vi "Periodic Tasks.vi"(8 "error in":errorcluster) -> (0 "error out":errorcluster)   [LabVIEW 2018]
doc: "This VI runs in parallel to other tasks. It can contain as many user-defined periodic loops as you need. These can carry out PID or other sorts of timed response."
uses:
  <vilib>/Rock Robotics/WPI/Joystick/WPI_JoystickDevRef.ctl
  <vilib>/Rock Robotics/WPI/Joystick/WPI_JoystickDeviceEnum.ctl
  <vilib>/Rock Robotics/WPI/RobotDrive/WPI_RobotDriveDevRef.ctl
  <vilib>/Rock Robotics/WPI/MotorControl/WPI_MotorControlDeviceRef.ctl
  <vilib>/Rock Robotics/WPI/MotorControl/WPI_MotorControlType.ctl
  <vilib>/Rock Robotics/SystemInterfaces/DIO/FPGA_DIOPWMChannel.ctl
  <vilib>/Rock Robotics/WPI/PWM/WPI_PWMDeadband.ctl
  <vilib>/Rock Robotics/SystemInterfaces/DIO/FPGA_DIOChannel.ctl
  <vilib>/Rock Robotics/WPI/Solenoid/WPI_SolenoidDevRef.ctl
  <vilib>/Rock Robotics/WPI/Solenoid/WPI_SolenoidChannel.ctl
  <vilib>/Rock Robotics/WPI/DigitalInput/WPI_DigitalInputDevRef.ctl
  Vision States.ctl
  <vilib>/Rock Robotics/WPI/DriverStation/WPI_DriverStationRobotMode2.ctl
  Hatch Retainer States.ctl
  HAB Bk Spd Motor States.ctl
  Hatch Kicking States.ctl
  <vilib>/Rock Robotics/WPI/Solenoid/WPI_SolenoidValue.ctl
  <vilib>/Rock Robotics/WPI/ThirdParty/Phoenix-LabVIEW/Motor Controller/Controls/CTRE_Phoenix_MotorControl_ControlMode.ctl
  <vilib>/Rock Robotics/WPI/ThirdParty/Phoenix-LabVIEW/Motor Controller/Controls/CTRE_Phoenix_MotorControl_MotionProfileTrajectoryPoint.ctl
  <vilib>/Rock Robotics/WPI/Utilities/WPI_GetSetVariantRefNum.vi
  <vilib>/Rock Robotics/WPI/ThirdParty/Phoenix-LabVIEW/Motor Controller/Get/CTRE_Phoenix_MotorController_GetQuadratureData.vi
  Robot Global Data.vi
  <vilib>/Rock Robotics/Network Tables/NT Write Boolean.vi
  <vilib>/Rock Robotics/WPI/Solenoid/WPI_SolenoidSetEnum.vi
  <vilib>/addons/control/pid/pid.llb/PID (DBL).vi
  <vilib>/Rock Robotics/Network Tables/NT Write Number.vi
  <vilib>/Rock Robotics/WPI/ThirdParty/Phoenix-LabVIEW/Motor Controller/Closed Loop/Motion Profile/CTRE_Phoenix_MotorControl_BufferedTrajectoryPointStream_WriteAll.vi
  <vilib>/Rock Robotics/Network Tables/NT Read Number.vi
  <vilib>/addons/control/pid/NI_PID_pid.lvlib
panel:
  in  "HAB3DriveModuleMotorDevRef 2":T1={"DeviceStatus"={"status"=FALSE, "code"=0, "source"=""}, "Type"=enum."PWM", "PWM"={"PWM Channel"=enum."Invalid", "DeadBand"={"Name"="", "maxPositivePwm"=0, "minPositivePwm"=0, "centerPwm"=0, "maxNegativePwm"=0, "minNegativePwm"=0, "angularRange"=0}}, "CAN"={"Device Number"=0, "SetOutput VI Ref"=variant(refnum<vi> refnum), "GetOutput VI Ref"=variant(refnum<vi> refnum), "Enable VI Ref"=variant(refnum<vi> refnum), "Disable VI Ref"=variant(refnum<vi> refnum), "Data"=variant}, "Invert"=FALSE, "DIO PWM"={"PWM \"Enable\" Channel"=enum."Invalid", "DIOChannel"=enum."Invalid", "PWM Rate"=0.0}}
  in  "BkSpdAdjusterMotorDevRef":T1={"DeviceStatus"={"status"=FALSE, "code"=0, "source"=""}, "Type"=enum."PWM", "PWM"={"PWM Channel"=enum."Invalid", "DeadBand"={"Name"="", "maxPositivePwm"=0, "minPositivePwm"=0, "centerPwm"=0, "maxNegativePwm"=0, "minNegativePwm"=0, "angularRange"=0}}, "CAN"={"Device Number"=0, "SetOutput VI Ref"=variant(refnum<vi> refnum), "GetOutput VI Ref"=variant(refnum<vi> refnum), "Enable VI Ref"=variant(refnum<vi> refnum), "Disable VI Ref"=variant(refnum<vi> refnum), "Data"=variant}, "Invert"=FALSE, "DIO PWM"={"PWM \"Enable\" Channel"=enum."Invalid", "DIOChannel"=enum."Invalid", "PWM Rate"=0.0}}
  in  "HABAssisterSolenoidDevRef":T6={"DevStatus"={"status"=FALSE, "code"=0, "source"=""}, "Pneumatics Control Module"=0, "Forward Solenoid Channel"=enum."Invalid", "Reverse Solenoid Channel"=enum."Invalid"}
  out "Right Traj. Pts Array":dbl[][](array[numeric])
  out "Left Traj. Pts Array":dbl[][](array[numeric])
  in  "Back HAB 3 Limit Switch":T8={"DevStatus"={"status"=FALSE, "code"=0, "source"=""}, "DIO Channel"=enum."Invalid"}
  in  "Front HAB 3 Limit Switch":T8={"DevStatus"={"status"=FALSE, "code"=0, "source"=""}, "DIO Channel"=enum."Invalid"}
  in  "BottomRetainerSwitchDevRef":T8={"DevStatus"={"status"=FALSE, "code"=0, "source"=""}, "DIO Channel"=enum."Invalid"}
  in  "TopRetainerSwitchDevRef":T8={"DevStatus"={"status"=FALSE, "code"=0, "source"=""}, "DIO Channel"=enum."Invalid"}
  in  "HatchRetainerMotorDevRef":T1={"DeviceStatus"={"status"=FALSE, "code"=0, "source"=""}, "Type"=enum."PWM", "PWM"={"PWM Channel"=enum."Invalid", "DeadBand"={"Name"="", "maxPositivePwm"=0, "minPositivePwm"=0, "centerPwm"=0, "maxNegativePwm"=0, "minNegativePwm"=0, "angularRange"=0}}, "CAN"={"Device Number"=0, "SetOutput VI Ref"=variant(refnum<vi> refnum), "GetOutput VI Ref"=variant(refnum<vi> refnum), "Enable VI Ref"=variant(refnum<vi> refnum), "Disable VI Ref"=variant(refnum<vi> refnum), "Data"=variant}, "Invert"=FALSE, "DIO PWM"={"PWM \"Enable\" Channel"=enum."Invalid", "DIOChannel"=enum."Invalid", "PWM Rate"=0.0}}
  in  "HAB3BackSolenoidDevRef":T6={"DevStatus"={"status"=FALSE, "code"=0, "source"=""}, "Pneumatics Control Module"=0, "Forward Solenoid Channel"=enum."Invalid", "Reverse Solenoid Channel"=enum."Invalid"}
  in  "HAB3FrontSolenoidDevRef":T6={"DevStatus"={"status"=FALSE, "code"=0, "source"=""}, "Pneumatics Control Module"=0, "Forward Solenoid Channel"=enum."Invalid", "Reverse Solenoid Channel"=enum."Invalid"}
  in  "AuxJoystickDevRef":T9={"Device"=enum."USB 1"}
  in  "DriveJoystickDevRef":T9={"Device"=enum."USB 1"}
  in  "HAB3DriveModuleMotorDevRef":T1={"DeviceStatus"={"status"=FALSE, "code"=0, "source"=""}, "Type"=enum."PWM", "PWM"={"PWM Channel"=enum."Invalid", "DeadBand"={"Name"="", "maxPositivePwm"=0, "minPositivePwm"=0, "centerPwm"=0, "maxNegativePwm"=0, "minNegativePwm"=0, "angularRange"=0}}, "CAN"={"Device Number"=0, "SetOutput VI Ref"=variant(refnum<vi> refnum), "GetOutput VI Ref"=variant(refnum<vi> refnum), "Enable VI Ref"=variant(refnum<vi> refnum), "Disable VI Ref"=variant(refnum<vi> refnum), "Data"=variant}, "Invert"=FALSE, "DIO PWM"={"PWM \"Enable\" Channel"=enum."Invalid", "DIOChannel"=enum."Invalid", "PWM Rate"=0.0}}
  in  "LifterSolenoidDevRef":T6={"DevStatus"={"status"=FALSE, "code"=0, "source"=""}, "Pneumatics Control Module"=0, "Forward Solenoid Channel"=enum."Invalid", "Reverse Solenoid Channel"=enum."Invalid"}
  in  "DriveJoystickDevRef":T9={"Device"=enum."USB 1"}
  in  "HatchCollectorMotorDevRef":T1={"DeviceStatus"={"status"=FALSE, "code"=0, "source"=""}, "Type"=enum."PWM", "PWM"={"PWM Channel"=enum."Invalid", "DeadBand"={"Name"="", "maxPositivePwm"=0, "minPositivePwm"=0, "centerPwm"=0, "maxNegativePwm"=0, "minNegativePwm"=0, "angularRange"=0}}, "CAN"={"Device Number"=0, "SetOutput VI Ref"=variant(refnum<vi> refnum), "GetOutput VI Ref"=variant(refnum<vi> refnum), "Enable VI Ref"=variant(refnum<vi> refnum), "Disable VI Ref"=variant(refnum<vi> refnum), "Data"=variant}, "Invert"=FALSE, "DIO PWM"={"PWM \"Enable\" Channel"=enum."Invalid", "DIOChannel"=enum."Invalid", "PWM Rate"=0.0}}
  in  "AuxJoystickDevRef":T9
  in  "RetainerSolenoidDevRef":T6={"DevStatus"={"status"=FALSE, "code"=0, "source"=""}, "Pneumatics Control Module"=0, "Forward Solenoid Channel"=enum."Invalid", "Reverse Solenoid Channel"=enum."Invalid"}
  in  "KickerSolenoidDevRef":T6={"DevStatus"={"status"=FALSE, "code"=0, "source"=""}, "Pneumatics Control Module"=0, "Forward Solenoid Channel"=enum."Invalid", "Reverse Solenoid Channel"=enum."Invalid"}
  in  "Drive Motors":T11={"DevStatus"={"status"=FALSE, "code"=0, "source"=""}, "Motors[]"=[], "Square Inputs"=FALSE, "Max Output"=1.0}
  in  "AuxJoystickDevRef":T9={"Device"=enum."USB 1"}
  in  "DriveJoystickDevRef":T9
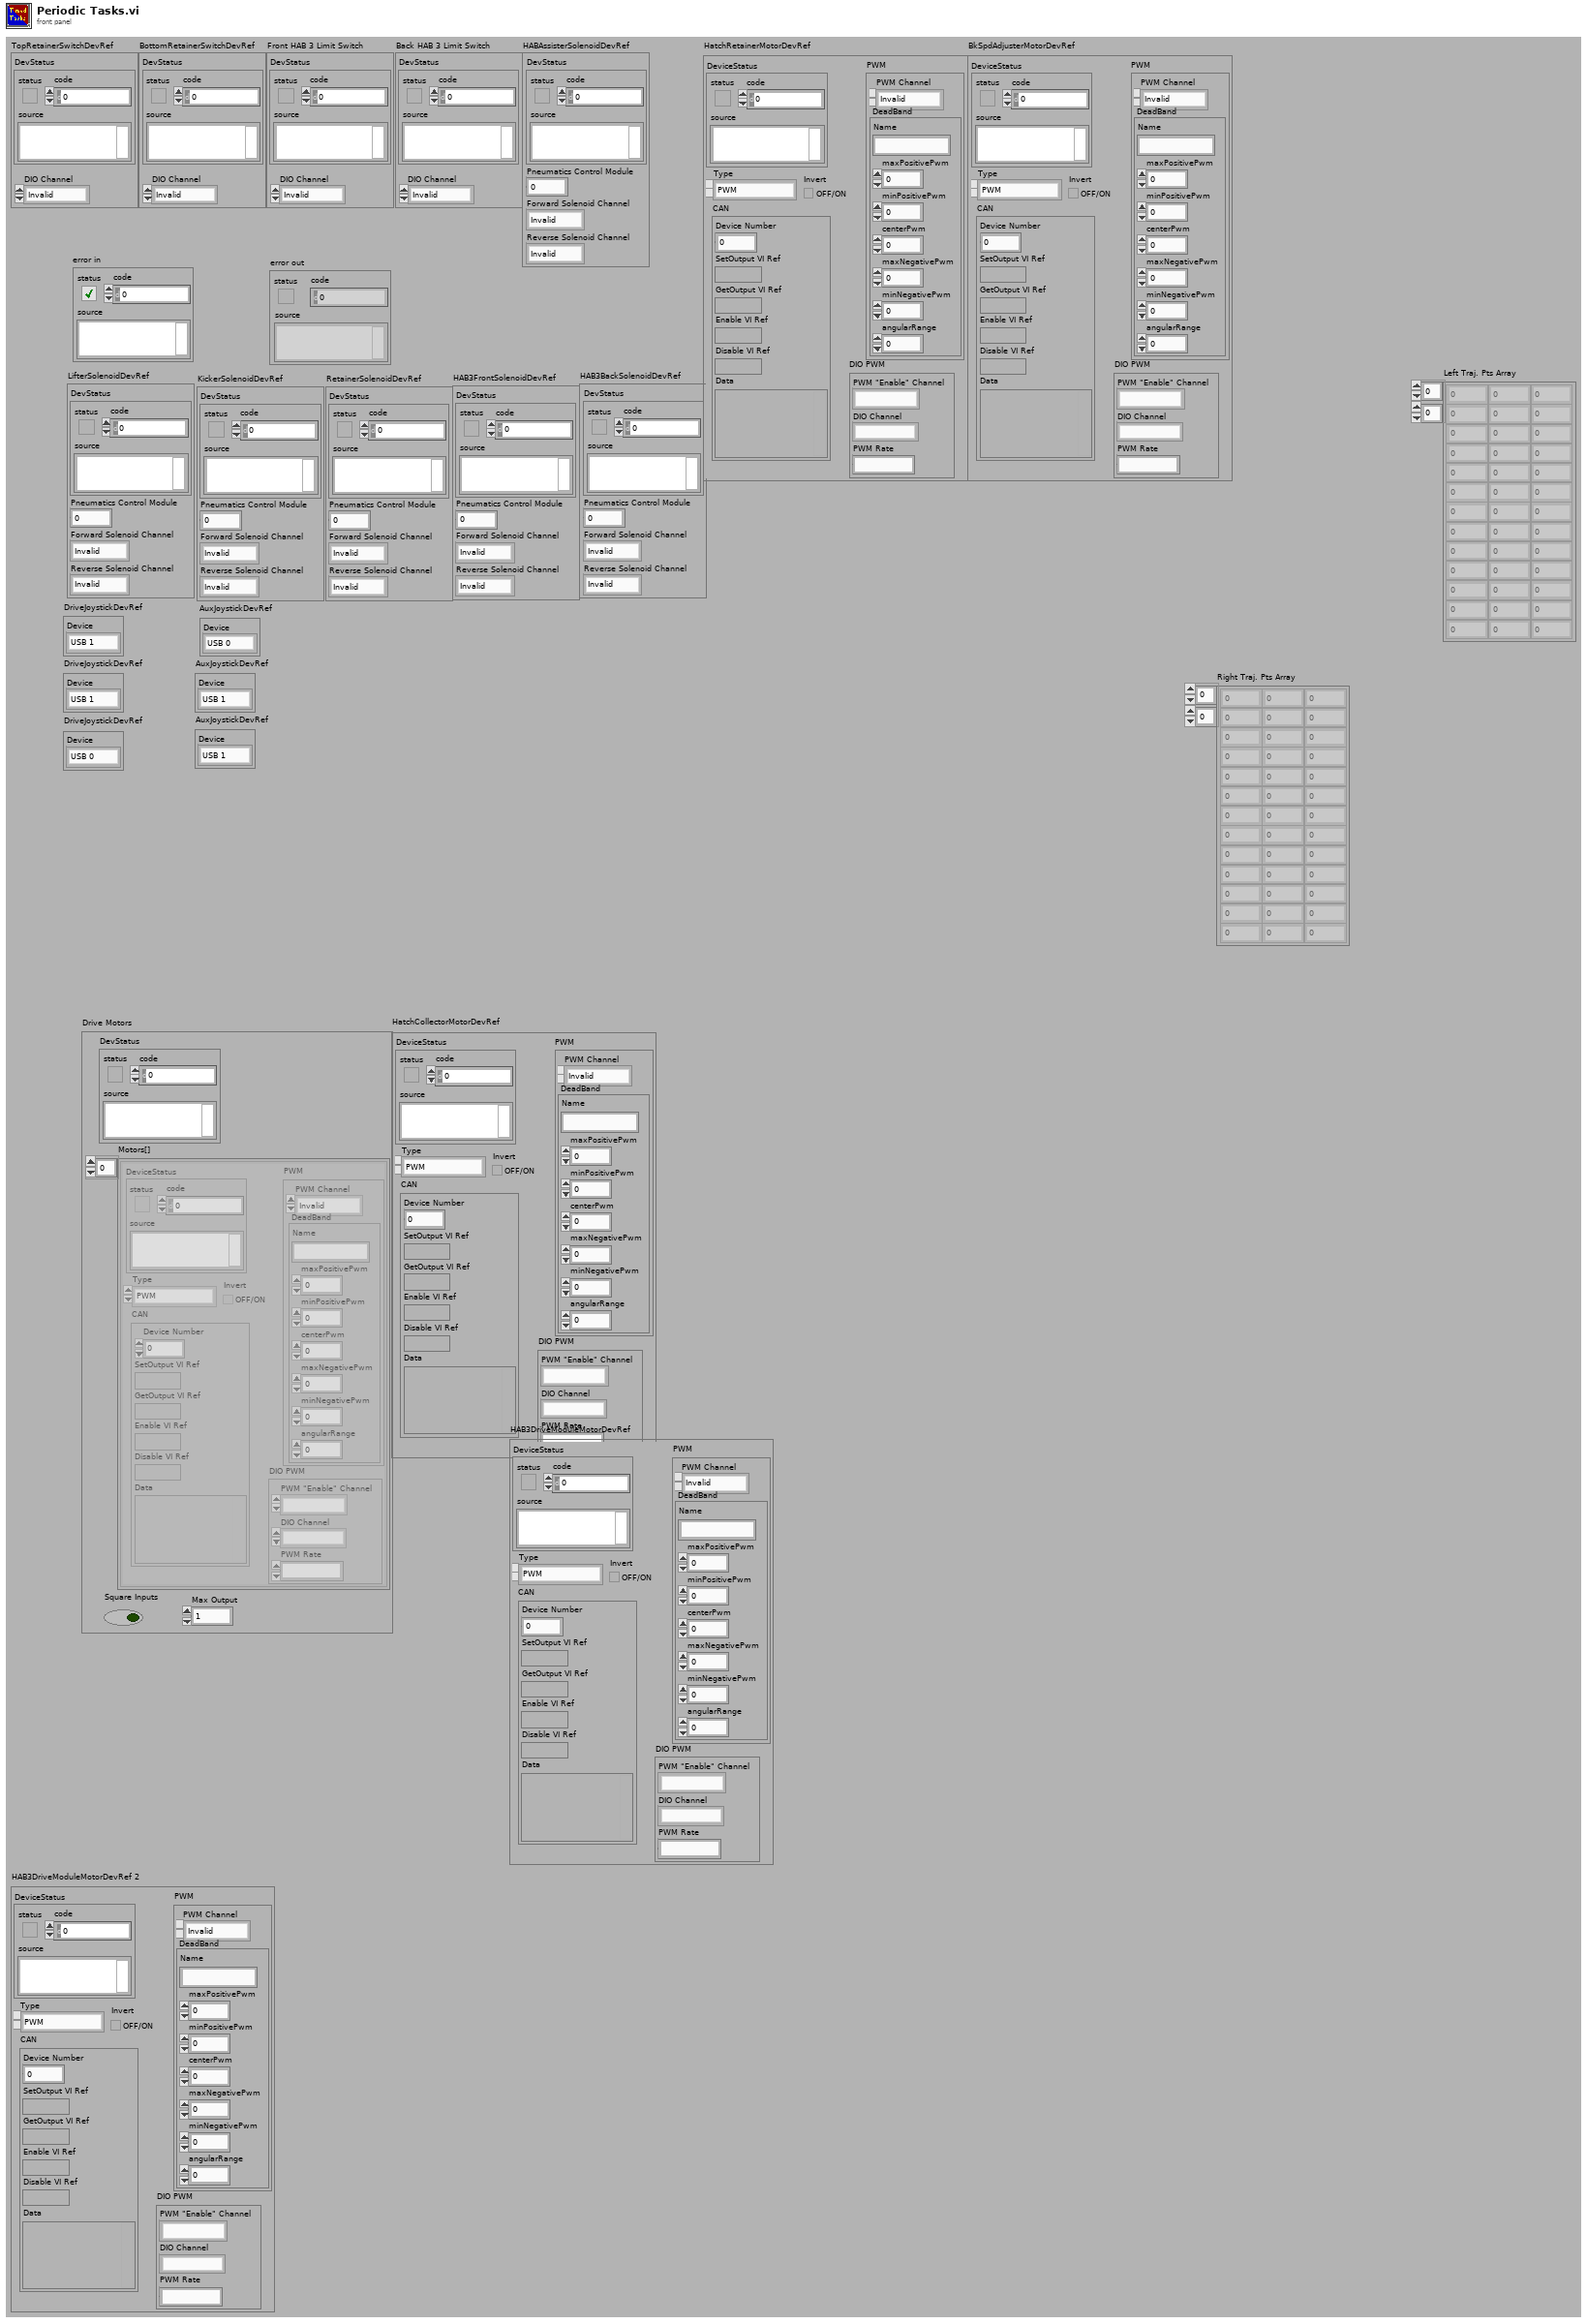
[diagram p1: front panel]
types:
  T1 = typedef "WPI_MotorControlDeviceRef.ctl" = cluster{"DeviceStatus":errorcluster, "Type":T2, "PWM":cluster{"PWM Channel":T3, "DeadBand":T4}, "CAN":cluster{"Device Number":u8, "SetOutput VI Ref":variant, "GetOutput VI Ref":variant, "Enable VI Ref":variant, "Disable VI Ref":variant, "Data":variant}, "Invert":bool, "DIO PWM":cluster{"PWM \"Enable\" Channel":T3, "DIOChannel":T5, "PWM Rate":dbl}}
  T2 = typedef "WPI_MotorControlType.ctl" = enum16{"PWM", "CAN", "DIO PWM"}
  T3 = typedef "FPGA_DIOPWMChannel.ctl" = enum8{"PWM 0", "PWM 1", "PWM 2", "PWM 3", "PWM 4", "PWM 5", "PWM 6", "PWM 7", "PWM 8", "PWM 9", "PWM MXP 0", "PWM MXP 1", "PWM MXP 2", "PWM MXP 3", "PWM MXP 4", "PWM MXP 5", "PWM MXP 6", "PWM MXP 7", "PWM MXP 8", "PWM MXP 9", "Invalid"}
  T4 = typedef "WPI_PWMDeadband.ctl" = cluster{"Name":string, "maxPositivePwm":i32, "minPositivePwm":i32, "centerPwm":i32, "maxNegativePwm":i32, "minNegativePwm":i32, "angularRange":u16}
  T5 = typedef "FPGA_DIOChannel.ctl" = enum8{"DIO 0", "DIO 1", "DIO 2", "DIO 3", "DIO 4", "DIO 5", "DIO 6", "DIO 7", "DIO 8", "DIO 9", "DIO MXP 0", "DIO MXP 1", "DIO MXP 2", "DIO MXP 3", "DIO MXP 4", "DIO MXP 5", "DIO MXP 6", "DIO MXP 7", "DIO MXP 8", "DIO MXP 9", "DIO MXP 10", "DIO MXP 11", "DIO MXP 12", "DIO MXP 13", "DIO MXP 14", "DIO MXP 15", "SPI Port CS1", "SPI Port CS2", "SPI Port CS3", "SPI Port MISO", "SPI Port MOSI", "Invalid"}
  T6 = typedef "WPI_SolenoidDevRef.ctl" = cluster{"DevStatus":errorcluster, "Pneumatics Control Module":u8, "Forward Solenoid Channel":T7, "Reverse Solenoid Channel":T7}
  T7 = typedef "WPI_SolenoidChannel.ctl" = enum8{"Solenoid 0", "Solenoid 1", "Solenoid 2", "Solenoid 3", "Solenoid 4", "Solenoid 5", "Solenoid 6", "Solenoid 7", "Invalid"}
  T8 = typedef "WPI_DigitalInputDevRef.ctl" = cluster{"DevStatus":errorcluster, "DIO Channel":T5}
  T9 = typedef "WPI_JoystickDevRef.ctl" = cluster{"Device":T10}
  T10 = typedef "WPI_JoystickDeviceEnum.ctl" = enum16{"USB 0", "USB 1", "USB 2", "USB 3", "USB 4", "USB 5"}
  T11 = typedef "WPI_RobotDriveDevRef.ctl" = cluster{"DevStatus":errorcluster, "Motors[]":T1[], "Square Inputs":bool, "Max Output":dbl}
  T12 = typedef "Hatch Kicking States.ctl" = enum16{"Ready", "Stop Retaining Hatch", "Kick Hatch"}
  T13 = typedef "HAB Bk Spd Motor States.ctl" = enum16{"Fully Up", "Going Down", "Fully Down", "Going Up"}
  T14 = typedef "Hatch Retainer States.ctl" = enum16{"Fully Down (not retained)", "Going Up", "Fully Up (retained)", "Going Down"}
  T15 = cluster{"X Button":i32, "A Button":i32, "B Button":i32, "Y Button":i32, "LB Button":i32, "RB Button":i32, "LT Button":i32, "RT Button":i32, "BACK Button":i32, "START Button":i32, "LJ Click Button":i32, "RJ Click Button":i32}
  T16 = cluster{"Left X":i32, "Left Y":i32, "Right X":i32, "Right Y":i32}
  T17 = typedef "WPI_DriverStationRobotMode2.ctl" = enum16{"Autonomous Disabled", "Autonomous Enabled", "Teleop Disabled", "Teleop Enabled", "Disconnected", "Finish", "Test Disabled", "Test Enabled", "Emergency Stopped"}
  T18 = cluster{"offsetAngle H":dbl, "offsetAngle V":dbl, "area":dbl, "skew":dbl, "shortest side (pxls)":dbl, "longest side (pxls)":dbl}
  T19 = typedef "Vision States.ctl" = enum16{"Ready", "Forward Until Target at Edge", "Vision Track"}
  T20 = cluster{"A Button":i32, "B Button":i32, "X Button":i32, "Y Button":i32, "LB Button":i32, "RB Button":i32, "BACK Button":i32, "START Button":i32, "LJ Click Button":i32, "RJ Click Button":i32}
  T21 = cluster{"Left X":i32, "Left Y":i32, "Right X":i32, "Right Y":i32, "RT Button":i32, "LT Button":i32}
  T22 = typedef "WPI_GyroDevRef.ctl" = cluster{"DevStatus":errorcluster, "Analog Channel":T23, "Gain (VoltsPerDegree/Second)":dbl, "Gyro Type":enum16{"Analog", "XRS450"}, "Handle":i32, "SPI Bus":T24, "Device Found":bool, "Sample Rate":dbl, "Calibrate On Open":bool, "Offset":dbl}
  T23 = typedef "FPGA_AIChannel.ctl" = enum8{"AI 0", "AI 1", "AI 2", "AI 3", "AI MXP 0", "AI MXP 1", "AI MXP 2", "AI MXP 3", "Invalid"}
  T24 = typedef "spi_bus.ctl" = enum16{"SPI On-Board, CS0", "SPI On-Board, CS1", "SPI On-Board, CS2", "SPI On-Board, CS3", "SPI MXP", "Invalid"}
  T25 = cluster{"HAB3DriveModuleMotorDevRef 2":T1, "DriveJoystickDevRef":T9, "AuxJoystickDevRef":T9, "Drive Axes":dbl[], "Drive Buttons":bool[], "Drive POVs":i16[], "Aux Axes":dbl[], "Aux Buttons":bool[], "Aux POVs":i16[], "Robot Mode":T17, "Drive Motors":T11, "Drive Axes Indexes":cluster{"Left X":i32, "Left Y":i32, "Right X":i32, "Right Y":i32, "RT Button":i32, "LT Button":i32}, "Drive Button Indexes":cluster{"A Button":i32, "B Button":i32, "X Button":i32, "Y Button":i32, "LB Button":i32, "RB Button":i32, "BACK Button":i32, "START Button":i32, "LJ Click Button":i32, "RJ Click Button":i32}, "Joystick VS Vision Latch":bool, "Vision States":T19, "limelight":cluster{"offsetAngle H":dbl, "offsetAngle V":dbl, "area":dbl, "skew":dbl, "shortest side (pxls)":dbl, "longest side (pxls)":dbl}, "Vision Track Mode Override":bool, "T = Motion Profile, F = Percent Output":bool, "Arcade Drive?":bool, "Start Motion Profile?":bool}
  T26 = cluster{"TopRetainerSwitchDevRef":T8, "BottomRetainerSwitchDevRef":T8, "HatchRetainerMotorDevRef":T1, "LifterSolenoidDevRef":T6, "DriveJoystickDevRef":T9, "KickerSolenoidDevRef":T6, "RetainerSolenoidDevRef":T6, "AuxJoystickDevRef":T9, "HatchCollectorMotorDevRef":T1, "Drive Axes":dbl[], "Drive Buttons":bool[], "Drive POVs":i16[], "Aux Axes":dbl[], "Aux Buttons":bool[], "Aux POVs":i16[], "Robot Mode":T17, "Aux Joystick Indexes":cluster{"Left X":i32, "Left Y":i32, "Right X":i32, "Right Y":i32}, "Aux Button Indexes":cluster{"X Button":i32, "A Button":i32, "B Button":i32, "Y Button":i32, "LB Button":i32, "RB Button":i32, "LT Button":i32, "RT Button":i32, "BACK Button":i32, "START Button":i32, "LJ Click Button":i32, "RJ Click Button":i32}, "Hatch Retainer Move Up/Down":bool, "Hatch Collector Actual Angle":dbl, "Hatch Collector Wanted Angle":dbl, "Hatch Retainer States":T14, "Hatch Kicking States":T12}
  T27 = cluster{"BkSpdAdjusterMotorDevRef":T1, "HABAssisterSolenoidDevRef":T6, "Back HAB 3 Limit Switch":T8, "Front HAB 3 Limit Switch":T8, "HAB3DriveModuleMotorDevRef":T1, "DriveJoystickDevRef":T9, "AuxJoystickDevRef":T9, "HAB3FrontSolenoidDevRef":T6, "HAB3BackSolenoidDevRef":T6, "Drive Axes":dbl[], "Drive Buttons":bool[], "Drive POVs":i16[], "Aux Axes":dbl[], "Aux Buttons":bool[], "Aux POVs":i16[], "Robot Mode":T17, "Aux Joystick Indexes":cluster{"Left X":i32, "Left Y":i32, "Right X":i32, "Right Y":i32}, "Aux Button Indexes":cluster{"X Button":i32, "A Button":i32, "B Button":i32, "Y Button":i32, "LB Button":i32, "RB Button":i32, "LT Button":i32, "RT Button":i32, "BACK Button":i32, "START Button":i32, "LJ Click Button":i32, "RJ Click Button":i32}, "Front Cylinders Latch":bool, "Back Cylinders Latch":bool, "Yaw":dbl, "Pitch":dbl, "Roll":dbl, "HAB Bk Spd Motor States":T13}
  T28 = typedef "CTRE_Phoenix_MotorControl_MotionProfileTrajectoryPoint.ctl" = cluster{"Position":dbl, "Velocity":dbl, "Arbitrary Feed Forward":dbl, "Auxiliary Position":dbl, "Auxiliary Velocity":dbl, "Auxiliary Arbitrary Feed Forward":dbl, "Profile Slot Select":i32, "Auxiliary Profile Slot Select":i32, "isLastPoint?":bool, "Zero Position?":bool, "durationMs":u32, "Use Aux PID?":bool}
  T29 = typedef "Which Robot Enum.ctl" = enum16{"Competition Bot", "Practice Bot", "Code Bot"}
  T30 = typedef "CTRE_Phoenix_MotorControl_BufferedTrajectoryPointStream_DeviceRef.ctl" = cluster{"Handle":u64, "Library Path":path}
  T31 = typedef "WPI_SolenoidValue.ctl" = enum16{"Off", "On", "Forward", "Reverse"}
  T32 = cluster{"proportional gain (Kc)":dbl, "integral time (Ti, min)":dbl, "derivative time (Td, min)":dbl}
  T33 = typedef "CTRE_Phoenix_MotorControl_ControlMode.ctl" = u16
  T34 = cluster{"Yaw":dbl, "Roll":dbl, "Pitch":dbl, "Heading":dbl, "Fused Heading":dbl}
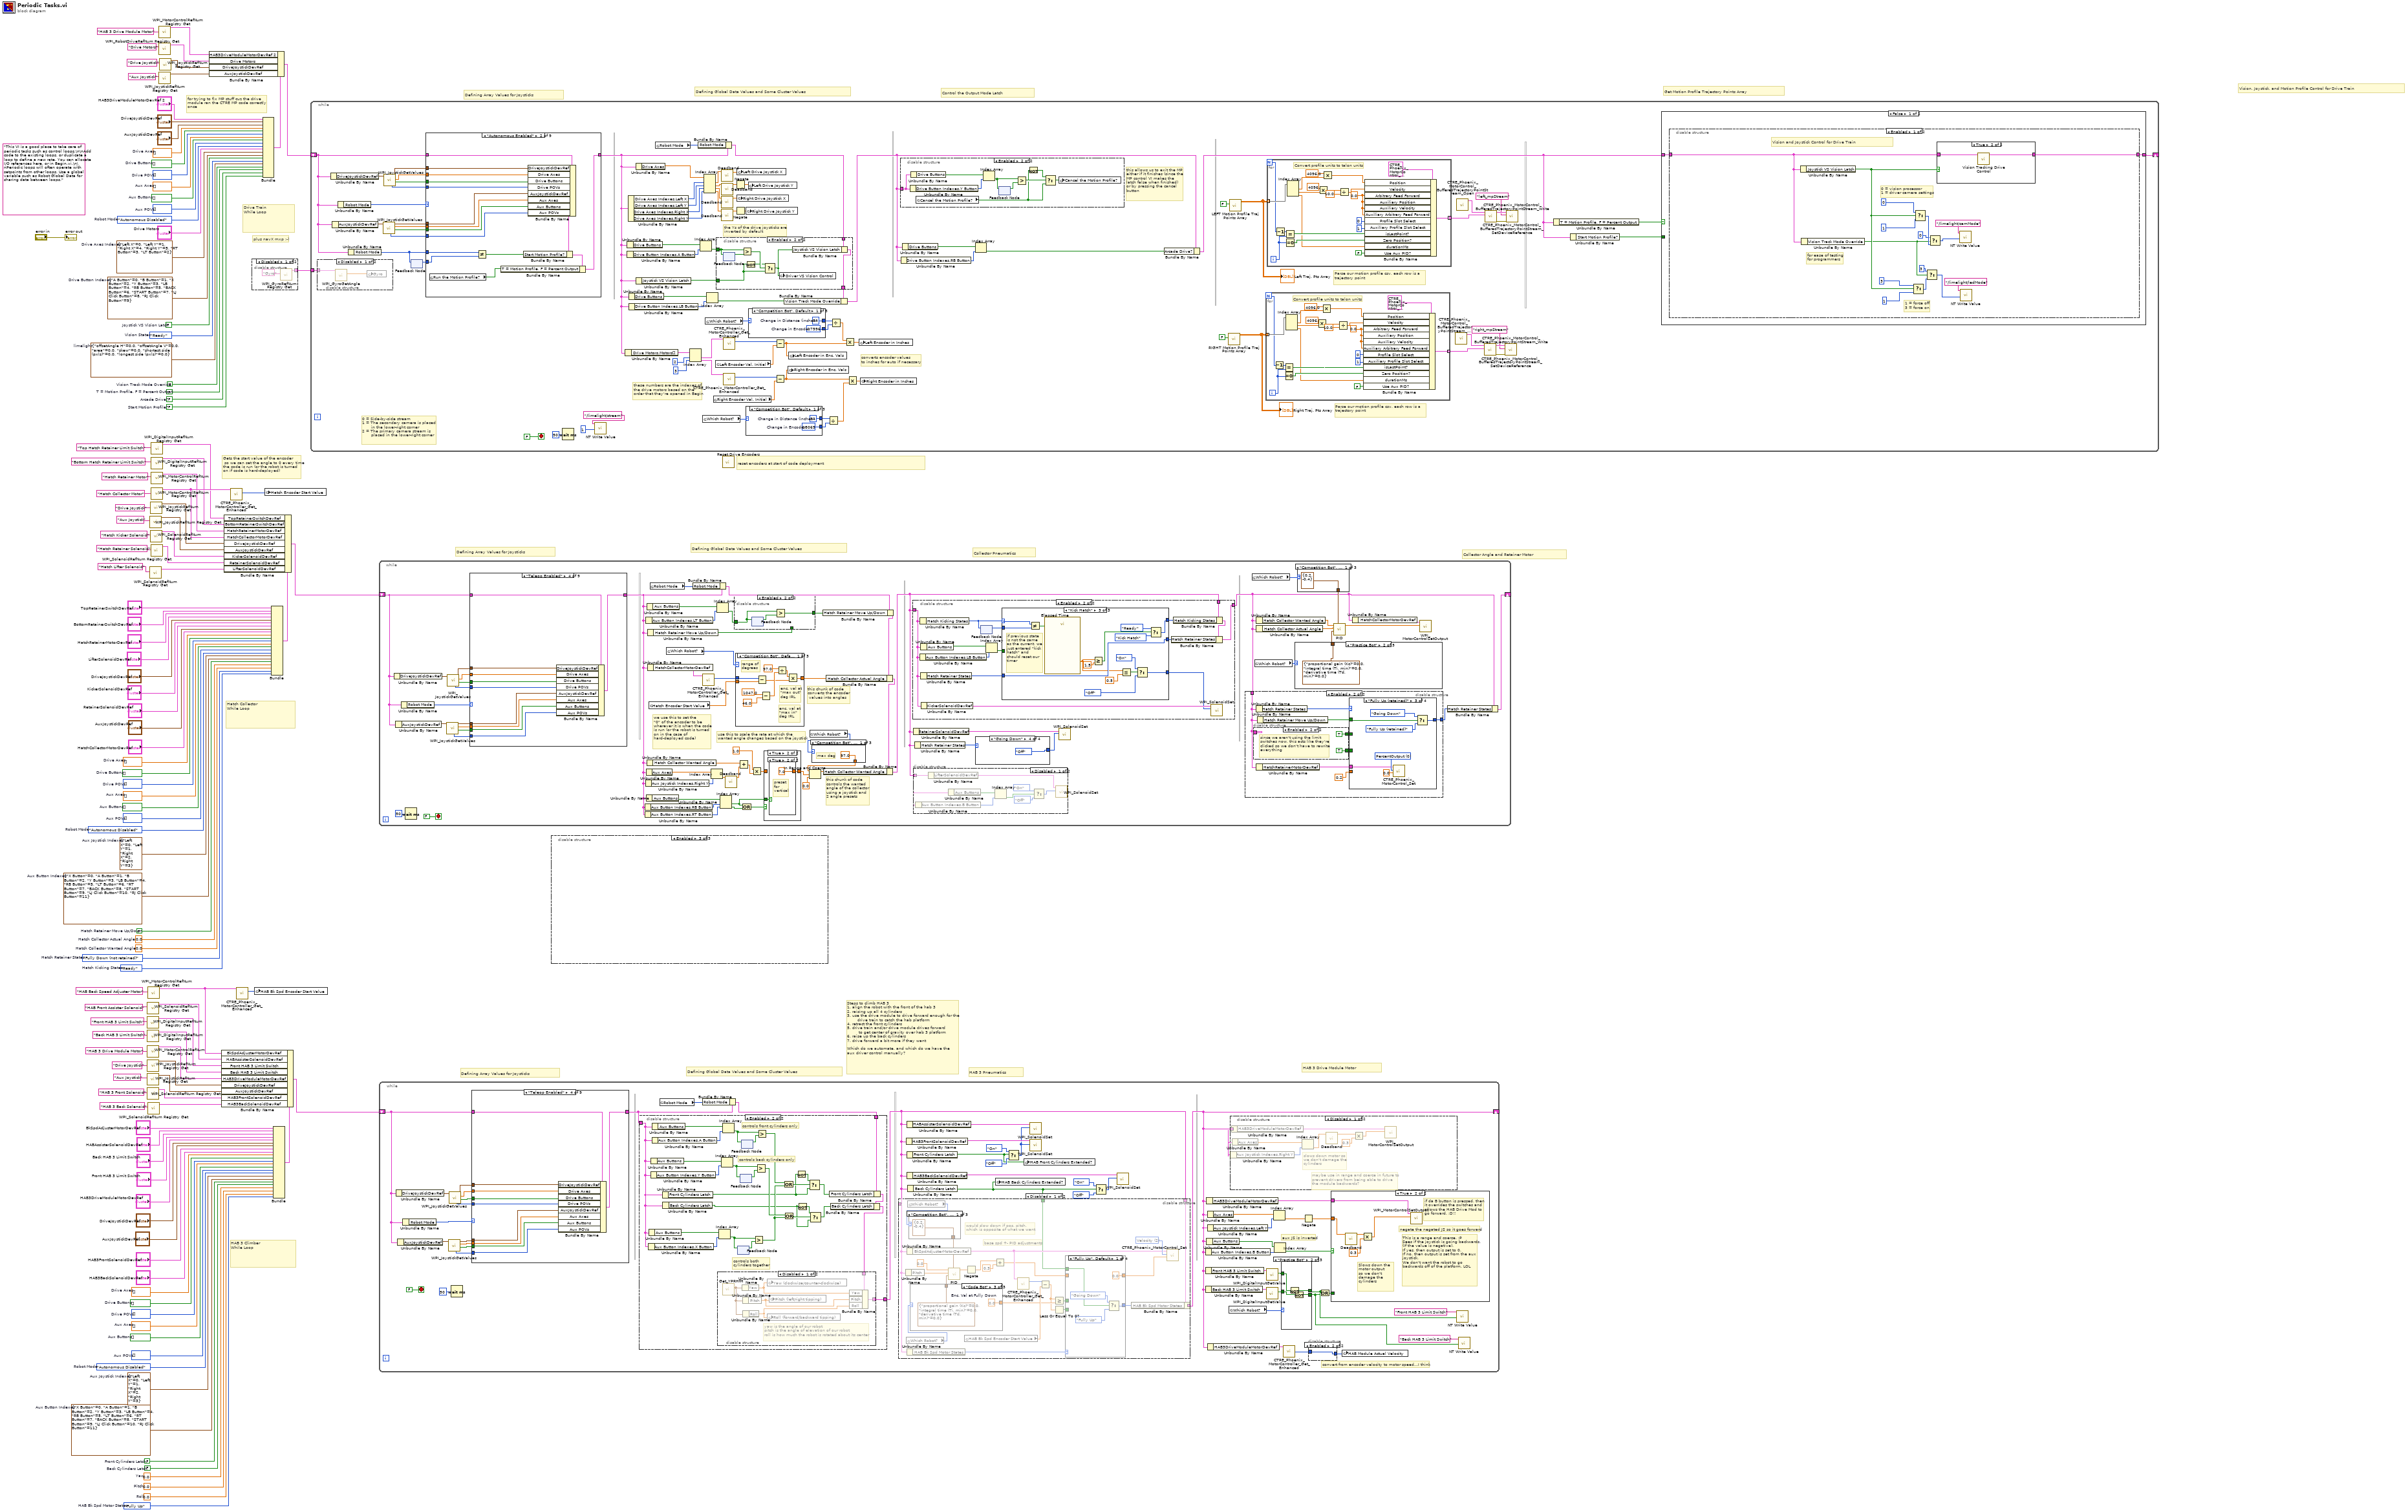
[diagram p0: block diagram]
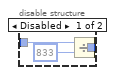
[diagram p2: hidden frame]
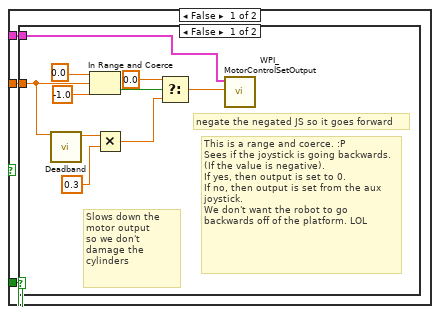
[diagram p3: hidden frame]
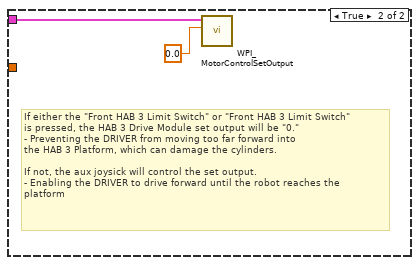
[diagram p4: hidden frame]
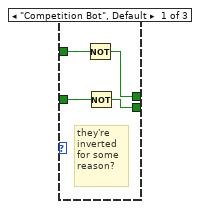
[diagram p5: hidden frame]
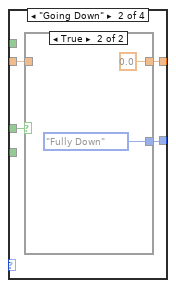
[diagram p7: hidden frame]
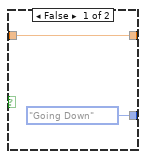
[diagram p8: hidden frame]
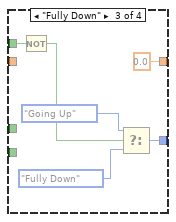
[diagram p9: hidden frame]
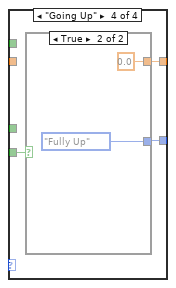
[diagram p10: hidden frame]
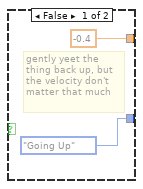
[diagram p11: hidden frame]
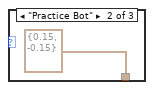
[diagram p12: hidden frame]
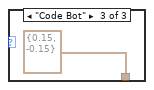
[diagram p13: hidden frame]
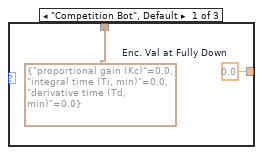
[diagram p14: hidden frame]
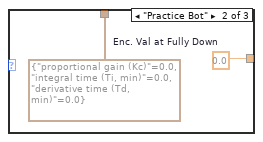
[diagram p15: hidden frame]
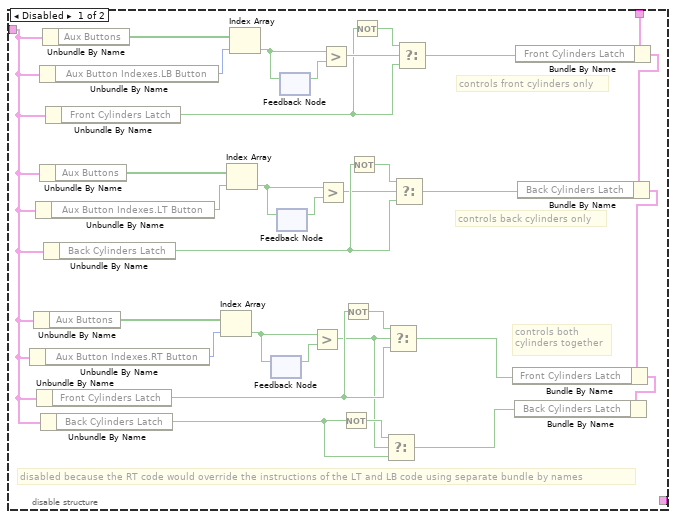
[diagram p17: hidden frame]
diagram:
  w4 = FALSE  # Start Motion Profile?
  w5 = FALSE  # Arcade Drive?
  w6 = Hatch_Kicking_States."Ready"  # Hatch Kicking States
  w7 = HAB_Bk_Spd_Motor_States."Fully Up"  # HAB Bk Spd Motor States
  w12 = 0.0  # Roll
  w13 = 0.0  # Pitch
  w14 = 0.0  # Yaw
  w24 = Hatch_Retainer_States."Fully Down (not retained)"  # Hatch Retainer States
  w34 = FALSE  # T = Motion Profile, F = Percent Output
  w36 = 0.0  # Hatch Collector Wanted Angle
  w37 = FALSE  # Back Cylinders Latch
  w38 = FALSE  # Front Cylinders Latch
  w39 = T15 {"X Button"=0, "A Button"=1, "B Button"=2, "Y Button"=3, "LB Button"=4, "RB Button"=5, "LT Button"=6, "RT Button"=7, "BACK Button"=8, "START Button"=9, "LJ Click Button"=10, "RJ Click Button"=11}  # Aux Button Indexes
  w40 = T16 {"Left X"=0, "Left Y"=1, "Right X"=2, "Right Y"=3}  # Aux Joystick Indexes
  w41 = WPI_DriverStationRobotMode2."Autonomous Disabled"  # Robot Mode
  w42 = i16[] []  # Aux POVs
  w43 = bool[] []  # Aux Buttons
  w44 = dbl[] []  # Aux Axes
  w45 = i16[] []  # Drive POVs
  w46 = bool[] []  # Drive Buttons
  w47 = dbl[] []  # Drive Axes
  w70 = 0.0  # Hatch Collector Actual Angle
  w71 = FALSE  # Hatch Retainer Move Up/Down
  w72 = T15 {"X Button"=0, "A Button"=1, "B Button"=2, "Y Button"=3, "LB Button"=4, "RB Button"=5, "LT Button"=6, "RT Button"=7, "BACK Button"=8, "START Button"=9, "LJ Click Button"=10, "RJ Click Button"=11}  # Aux Button Indexes
  w73 = T16 {"Left X"=0, "Left Y"=1, "Right X"=2, "Right Y"=3}  # Aux Joystick Indexes
  w77 = WPI_DriverStationRobotMode2."Autonomous Disabled"  # Robot Mode
  w78 = i16[] []  # Aux POVs
  w79 = bool[] []  # Aux Buttons
  w80 = dbl[] []  # Aux Axes
  w81 = i16[] []  # Drive POVs
  w82 = bool[] []  # Drive Buttons
  w83 = dbl[] []  # Drive Axes
  w97 = FALSE  # Vision Track Mode Override
  w98 = T18 {"offsetAngle H"=0.0, "offsetAngle V"=0.0, "area"=0.0, "skew"=0.0, "shortest side (pxls)"=0.0, "longest side (pxls)"=0.0}  # limelight
  w99 = Vision_States."Ready"  # Vision States
  w100 = FALSE  # Joystick VS Vision Latch
  w101 = T20 {"A Button"=0, "B Button"=1, "X Button"=2, "Y Button"=3, "LB Button"=4, "RB Button"=5, "BACK Button"=6, "START Button"=7, "LJ Click Button"=8, "RJ Click Button"=9}  # Drive Button Indexes
  w103 = T21 {"Left X"=0, "Left Y"=1, "Right X"=4, "Right Y"=5, "RT Button"=3, "LT Button"=2}  # Drive Axes Indexes
  w108 = i16[] []  # Aux POVs
  w109 = bool[] []  # Aux Buttons
  w110 = dbl[] []  # Aux Axes
  w107 = WPI_DriverStationRobotMode2."Autonomous Disabled"  # Robot Mode
  w111 = i16[] []  # Drive POVs
  w112 = bool[] []  # Drive Buttons
  w113 = dbl[] []  # Drive Axes
  (unwired) "This VI is a good place to take care of periodic tasks such as control loops.\n\nAdd code to the existing loops, or duplicate a loop to define a new rate. You can allocate I/O references here, or in Begin.vi.\n\nPeriodic loops will often operate with setpoints from other loops. Use a global variable such as Robot Global Data for sharing data between loops."
  # "HAB 3 Drive Module Motor"
  # "HAB 3 Pneumatics"
  # "Steps to climb HAB 3\n1. align the robot with the front of the hab 3\n2. raising up all 4 cylinders\n3. use the drive module to drive forward enough for the \n        drive train to catch the hab platform\n4. retract the front cylinders\n5. drive train and/or drive module drives forward \n         to get center of gravity over hab 3 platform\n6. raise up the back cylinders\n7. drive forward a bit more if they want\n\nWhich do we automate, and which do we have the \naux driver control manually?"
  # "Defining Global Data Values and Some Cluster Values"
  # "Defining Array Values for Joysticks"
  # "Collector Angle and Retainer Motor"
  # "Collector Pneumatics"
  # "Defining Global Data Values and Some Cluster Values"
  # "Defining Array Values for Joysticks"
  # "for trying to fix MP stuff cuz the drive\nmodule ran the CTRE MP code correctly\nonce"
  # "reset encoders at start of code deployment"
  # "Get Motion Profile Trajectory Points Array"
  # "Control the Output Mode Latch"
  # "plus navX mxp :-)"
  # "Gets the start value of the encoder\n so we can set the angle to 0 every time\nthe code is run (or the robot is turned\non if code is hard-deployed)"
  # "HAB 3 Climber\nWhile Loop"
  # "Hatch Collector\nWhile Loop"
  # "Drive Train\nWhile Loop"
  # "Vision, Joystick, and Motion Profile Control for Drive Train"
  # "Defining Array Values for Joysticks"
  # "Defining Global Data Values and Some Cluster Values"
  n1 = call <vilib>:"WPI_DigitalInputRefNum Registry Get.vi"("refnum name"="Front HAB 3 Limit Switch") -> ("DigitalInputDevRef"=w19:T8)  [unwired: 9 in, 1 out]
  n2 = call <vilib>:"WPI_JoystickRefNum Registry Get.vi"("refnum name"="Aux Joystick") -> ("JoystickDevRef"=w51:T9)  [unwired: 9 in, 1 out]
  n3 = call <vilib>:"WPI_SolenoidRefNum Registry Get.vi"("refnum name"="HAB Front Assister Solenoid") -> ("SolenoidDevRef"=w15:T6)  [unwired: 9 in, 1 out]
  n4 = call <vilib>:"WPI_DigitalInputRefNum Registry Get.vi"("refnum name"="Back HAB 3 Limit Switch") -> ("DigitalInputDevRef"=w18:T8)  [unwired: 9 in, 1 out]
  n5 = call <vilib>:"WPI_MotorControlRefNum Registry Get.vi"("refnum name"="HAB 3 Drive Module Motor") -> ("MotorControlDevRef"=w49:T1)  [unwired: 9 in, 1 out]
  n6 = call <vilib>:"WPI_JoystickRefNum Registry Get.vi"("refnum name"="Drive Joystick") -> ("JoystickDevRef"=w50:T9)  [unwired: 9 in, 1 out]
  n7 = call <vilib>:"WPI_SolenoidRefNum Registry Get.vi"("refnum name"="HAB 3 Front Solenoid") -> ("SolenoidDevRef"=w52:T6)  [unwired: 9 in, 1 out]
  n8 = call <vilib>:"WPI_MotorControlRefNum Registry Get.vi"("refnum name"="HAB Back Speed Adjuster Motor") -> ("MotorControlDevRef"=w8:T1)  [unwired: 9 in, 1 out]
  n9 = call <vilib>:"WPI_SolenoidRefNum Registry Get.vi"("refnum name"="HAB 3 Back Solenoid") -> ("SolenoidDevRef"=w53:T6)  [unwired: 9 in, 1 out]
  n10 = call <vilib>:"WPI_SolenoidRefNum Registry Get.vi"("refnum name"="Hatch Lifter Solenoid") -> ("SolenoidDevRef"=w66:T6)  [unwired: 9 in, 1 out]
  n11 = call <vilib>:"WPI_JoystickRefNum Registry Get.vi"("refnum name"="Aux Joystick") -> ("JoystickDevRef"=w88:T9)  [unwired: 9 in, 1 out]
  n12 = call <vilib>:"WPI_JoystickRefNum Registry Get.vi"("refnum name"="Drive Joystick") -> ("JoystickDevRef"=w74:T9)  [unwired: 9 in, 1 out]
  n13 = call <vilib>:"WPI_SolenoidRefNum Registry Get.vi"("refnum name"="Hatch Kicker Solenoid") -> ("SolenoidDevRef"=w91:T6)  [unwired: 9 in, 1 out]
  n14 = call <vilib>:"WPI_SolenoidRefNum Registry Get.vi"("refnum name"="Hatch Retainer Solenoid") -> ("SolenoidDevRef"=w90:T6)  [unwired: 9 in, 1 out]
  n15 = call <vilib>:"WPI_DigitalInputRefNum Registry Get.vi"("refnum name"="Top Hatch Retainer Limit Switch") -> ("DigitalInputDevRef"=w25:T8)  [unwired: 9 in, 1 out]
  n16 = call <vilib>:"WPI_DigitalInputRefNum Registry Get.vi"("refnum name"="Bottom Hatch Retainer Limit Switch") -> ("DigitalInputDevRef"=w26:T8)  [unwired: 9 in, 1 out]
  n17 = call <vilib>:"WPI_MotorControlRefNum Registry Get.vi"("refnum name"="Hatch Retainer Motor") -> ("MotorControlDevRef"=w31:T1)  [unwired: 9 in, 1 out]
  n18 = call <vilib>:"WPI_MotorControlRefNum Registry Get.vi"("refnum name"="Hatch Collector Motor") -> ("MotorControlDevRef"=w69:T1)  [unwired: 9 in, 1 out]
  n19 = call <vilib>:"WPI_MotorControlRefNum Registry Get.vi"("refnum name"="HAB 3 Drive Module Motor") -> ("MotorControlDevRef"=w1:T1)  [unwired: 9 in, 1 out]
  n20 = call <vilib>:"WPI_RobotDriveRefNum Registry Get.vi"("refnum name"="Drive Motors") -> ("RobotDriveDevRef"=w105:T11)  [unwired: 9 in, 1 out]
  n21 = call <vilib>:"WPI_JoystickRefNum Registry Get.vi"("refnum name"="Aux Joystick") -> ("JoystickDevRef"=w115:T9)  [unwired: 9 in, 1 out]
  n22 = call <vilib>:"WPI_JoystickRefNum Registry Get.vi"("refnum name"="Drive Joystick") -> ("JoystickDevRef"=w116:T9)  [unwired: 9 in, 1 out]
  n23 = call-poly <vilib>:"CTRE_Phoenix_MotorController_Get_Enhanced.vi"("PhoenixMotorControlDevRef"=w69) -> ("Quadrature Position"=w68:i32)  [unwired: 11 in, 3 out]
  n24 = call-poly <vilib>:"CTRE_Phoenix_MotorController_Get_Enhanced.vi"("PhoenixMotorControlDevRef"=w8) -> ("Quadrature Position"=w9:i32)  [unwired: 11 in, 3 out]
  n25 = disable-structure shown="Disabled" {
    disable-tunnel: [w122 _] -> w35
    frame Disabled {
      n26 = call <vilib>:"WPI_GyroRefNum Registry Get.vi"("refnum name"="Gyro") -> ("GyroDevRef"=w122:T22)  [unwired: 9 in, 1 out]
    }
    frame Enabled {
    }
  }
  n27 = global write "Robot Global Data.vi" "HAB Bk Spd Encoder Start Value"(w9) -> ()
  n28 = Bundle("HAB3DriveModuleMotorDevRef 2"="HAB3DriveModuleMotorDevRef 2", "DriveJoystickDevRef"="DriveJoystickDevRef", "AuxJoystickDevRef"="AuxJoystickDevRef", "Drive Axes"=w113, "Drive Buttons"=w112, "Drive POVs"=w111, "Aux Axes"=w110, "Aux Buttons"=w109, "Aux POVs"=w108, "Robot Mode"=w107, "Drive Motors"="Drive Motors", "Drive Axes Indexes"=w103, "Drive Button Indexes"=w101, "Joystick VS Vision Latch"=w100, "Vision States"=w99, "limelight"=w98, "Vision Track Mode Override"=w97, "T = Motion Profile, F = Percent Output"=w34, "Arcade Drive?"=w5, "Start Motion Profile?"=w4) -> (w117:T25)  [unwired: 1 in]
  n29 = Bundle By Name(cluster=w117, "HAB3DriveModuleMotorDevRef 2"=w1, "Drive Motors"=w105, "DriveJoystickDevRef"=w116, "AuxJoystickDevRef"=w115) -> (w114:T25)
  n30 = global write "Robot Global Data.vi" "Hatch Encoder Start Value"(w68) -> ()
  n31 = Bundle("TopRetainerSwitchDevRef"="TopRetainerSwitchDevRef", "BottomRetainerSwitchDevRef"="BottomRetainerSwitchDevRef", "HatchRetainerMotorDevRef"="HatchRetainerMotorDevRef", "LifterSolenoidDevRef"="LifterSolenoidDevRef", "DriveJoystickDevRef"="DriveJoystickDevRef", "KickerSolenoidDevRef"="KickerSolenoidDevRef", "RetainerSolenoidDevRef"="RetainerSolenoidDevRef", "AuxJoystickDevRef"="AuxJoystickDevRef", "HatchCollectorMotorDevRef"="HatchCollectorMotorDevRef", "Drive Axes"=w83, "Drive Buttons"=w82, "Drive POVs"=w81, "Aux Axes"=w80, "Aux Buttons"=w79, "Aux POVs"=w78, "Robot Mode"=w77, "Aux Joystick Indexes"=w73, "Aux Button Indexes"=w72, "Hatch Retainer Move Up/Down"=w71, "Hatch Collector Actual Angle"=w70, "Hatch Collector Wanted Angle"=w36, "Hatch Retainer States"=w24, "Hatch Kicking States"=w6) -> (w94:T26)  [unwired: 1 in]
  n32 = Bundle By Name(cluster=w94, "TopRetainerSwitchDevRef"=w25, "BottomRetainerSwitchDevRef"=w26, "HatchRetainerMotorDevRef"=w31, "HatchCollectorMotorDevRef"=w69, "DriveJoystickDevRef"=w74, "AuxJoystickDevRef"=w88, "KickerSolenoidDevRef"=w91, "RetainerSolenoidDevRef"=w90, "LifterSolenoidDevRef"=w66) -> (w84:T26)
  n33 = Bundle("BkSpdAdjusterMotorDevRef"="BkSpdAdjusterMotorDevRef", "HABAssisterSolenoidDevRef"="HABAssisterSolenoidDevRef", "Back HAB 3 Limit Switch"="Back HAB 3 Limit Switch", "Front HAB 3 Limit Switch"="Front HAB 3 Limit Switch", "HAB3DriveModuleMotorDevRef"="HAB3DriveModuleMotorDevRef", "DriveJoystickDevRef"="DriveJoystickDevRef", "AuxJoystickDevRef"="AuxJoystickDevRef", "HAB3FrontSolenoidDevRef"="HAB3FrontSolenoidDevRef", "HAB3BackSolenoidDevRef"="HAB3BackSolenoidDevRef", "Drive Axes"=w47, "Drive Buttons"=w46, "Drive POVs"=w45, "Aux Axes"=w44, "Aux Buttons"=w43, "Aux POVs"=w42, "Robot Mode"=w41, "Aux Joystick Indexes"=w40, "Aux Button Indexes"=w39, "Front Cylinders Latch"=w38, "Back Cylinders Latch"=w37, "Yaw"=w14, "Pitch"=w13, "Roll"=w12, "HAB Bk Spd Motor States"=w7) -> (w54:T27)  [unwired: 1 in]
  n34 = Bundle By Name(cluster=w54, "BkSpdAdjusterMotorDevRef"=w8, "HABAssisterSolenoidDevRef"=w15, "Front HAB 3 Limit Switch"=w19, "Back HAB 3 Limit Switch"=w18, "HAB3DriveModuleMotorDevRef"=w49, "DriveJoystickDevRef"=w50, "AuxJoystickDevRef"=w51, "HAB3FrontSolenoidDevRef"=w52, "HAB3BackSolenoidDevRef"=w53) -> (w48:T27)
  n35 = while {
    shift-right: [w210] -> _
    shift-left: w114 -> [w129]
    tunnel: w35 -> [w172]
    stop <- FALSE stop-if-true
    # "0 = Side-by-side stream\n1 = The secondary camera is placed\n       in the lower-right corner\n2 = The primary camera stream is\n       placed in the lower-right corner"
    # "converts encoder values\nto inches for auto if necessary"
    # "Parse our motion profile csv, each row is a trajectory point"
    # "Parse our motion profile csv, each row is a trajectory point"
    # "this allows us to exit the MP \neither if it finishes (since the\nMP control VI makes the\nlatch false when finished) \nor by pressing the cancel \nbutton"
    # "these numbers are the indexes of\nthe drive motors based on the\norder that they're opened in Begin"
    # "the Ys of the drive joysticks are \ninverted by default"
    n36 = disable-structure shown="Disabled" {
      disable-tunnel: w172 -> [w378 _]
      frame Disabled {
        n37 = call <vilib>:"WPI_GyroGetAngle.vi"("GyroDevRef"=w378) -> ("Angle"=w379:dbl)  [unwired: 6 in, 4 out]
        n38 = global write "Robot Global Data.vi" "Gyro"(w379) -> ()
      }
      frame Enabled {
      }
    }
    n39 = Unbundle By Name(w129) -> ("DriveJoystickDevRef"=w208:T9)
    n40 = Unbundle By Name(w129) -> ("AuxJoystickDevRef"=w207:T9)
    n41 = Unbundle By Name(w129) -> ("Robot Mode"=w206:T17)
    n42 = Unbundle By Name(w129) -> ("Robot Mode"=w128:T17)
    n43 = call <vilib>:"WPI_JoystickGetValues.vi"("JoystickDevRef"=w207) -> ("Buttons"=w199:bool[], "Axes"=w200:dbl[], "JoystickDevRef"=w201:T9, "POVs"=w198:i16[])  [unwired: 6 in, 1 out]
    n44 = call <vilib>:"WPI_JoystickGetValues.vi"("JoystickDevRef"=w208) -> ("Buttons"=w203:bool[], "Axes"=w205:dbl[], "JoystickDevRef"=w204:T9, "POVs"=w202:i16[])  [unwired: 6 in, 1 out]
    n45 = feedback #1() -> (w127:T17)  [unwired: 1 in]
    n46 = feedback-in #1(w128) -> ()
    n47 = case shown="\"Autonomous Enabled\"" w206 {
      tunnel: w129 -> [w396 w418 w424 w444 w450 w462 w474 w494 w500]
      tunnel: [w392 w404 w419 w431 w445 w457 w469 w481 w495] -> w171
      tunnel: w205 -> [_ w417 _ w442 _ _ _ w492 _]
      tunnel: w204 -> [_ w416 _ w443 _ _ _ w493 _]
      tunnel: w203 -> [_ w415 _ w441 _ _ _ w491 _]
      tunnel: w202 -> [_ w414 _ w440 _ _ _ w490 _]
      tunnel: w201 -> [_ w413 _ w439 _ _ _ w489 _]
      tunnel: w200 -> [_ w412 _ w438 _ _ _ w488 _]
      tunnel: w199 -> [_ w411 _ w437 _ _ _ w487 _]
      tunnel: w198 -> [_ w410 _ w436 _ _ _ w486 _]
      tunnel: w128 -> [_ w409 _ _ _ _ _ _ _]
      tunnel: w127 -> [_ w408 _ _ _ _ _ _ _]
      frame "Autonomous Disabled", Default {
        n48 = disable-structure shown="Enabled" {
          disable-tunnel: w396 -> [w398 w402]
          disable-tunnel: [w397 w401] -> w394
          frame Disabled {
            n49 = Bundle By Name(cluster=w398, "Joystick VS Vision Latch"=FALSE) -> (w397:T25)
          }
          frame Enabled {
            n50 = Bundle By Name(cluster=w402, "Vision States"=Vision_States."Ready") -> (w401:T25)
          }
        }
        n51 = Bundle By Name(cluster=w394, "Start Motion Profile?"=FALSE ("T = Motion Profile, F = Percent Output")) -> (w393:T25)
        n52 = Bundle By Name(cluster=w393, "T = Motion Profile, F = Percent Output"=FALSE) -> (w392:T25)
      }
      frame "Autonomous Enabled" {
        n53 = global read "Robot Global Data.vi" "Run the Motion Profile?"() -> (w403:bool)
        n54 = Not Equal?(x=w409, y=w408) -> (x != y?=w407:bool)
        n55 = Bundle By Name(cluster=w418, "DriveJoystickDevRef"=w416, "Drive Axes"=w417, "Drive Buttons"=w415, "Drive POVs"=w414, "AuxJoystickDevRef"=w413, "Aux Axes"=w412, "Aux Buttons"=w411, "Aux POVs"=w410) -> (w406:T25)
        n56 = Bundle By Name(cluster=w406, "Start Motion Profile?"=w407) -> (w405:T25)
        n57 = Bundle By Name(cluster=w405, "T = Motion Profile, F = Percent Output"=w403) -> (w404:T25)
      }
      frame "Teleop Disabled" {
        n58 = disable-structure shown="Enabled" {
          disable-tunnel: w424 -> [w426 w430]
          disable-tunnel: [w425 w429] -> w422
          frame Disabled {
            n59 = Bundle By Name(cluster=w426, "Joystick VS Vision Latch"=FALSE) -> (w425:T25)
          }
          frame Enabled {
            n60 = Bundle By Name(cluster=w430, "Vision States"=Vision_States."Ready") -> (w429:T25)
          }
        }
        n61 = Bundle By Name(cluster=w422, "Start Motion Profile?"=FALSE ("T = Motion Profile, F = Percent Output")) -> (w420:T25)
        n62 = Bundle By Name(cluster=w420, "T = Motion Profile, F = Percent Output"=FALSE) -> (w419:T25)
      }
      frame "Teleop Enabled" {
        n63 = Bundle By Name(cluster=w444, "DriveJoystickDevRef"=w443, "Drive Axes"=w442, "Drive Buttons"=w441, "Drive POVs"=w440, "AuxJoystickDevRef"=w439, "Aux Axes"=w438, "Aux Buttons"=w437, "Aux POVs"=w436) -> (w435:T25)
        n64 = Bundle By Name(cluster=w435, "Start Motion Profile?"=FALSE ("T = Motion Profile, F = Percent Output")) -> (w432:T25)
        n65 = Bundle By Name(cluster=w432, "T = Motion Profile, F = Percent Output"=FALSE) -> (w431:T25)
      }
      frame "Disconnected" {
        n66 = disable-structure shown="Enabled" {
          disable-tunnel: w450 -> [w452 w456]
          disable-tunnel: [w451 w455] -> w448
          frame Disabled {
            n67 = Bundle By Name(cluster=w452, "Joystick VS Vision Latch"=FALSE) -> (w451:T25)
          }
          frame Enabled {
            n68 = Bundle By Name(cluster=w456, "Vision States"=Vision_States."Ready") -> (w455:T25)
          }
        }
        n69 = Bundle By Name(cluster=w448, "Start Motion Profile?"=FALSE ("T = Motion Profile, F = Percent Output")) -> (w446:T25)
        n70 = Bundle By Name(cluster=w446, "T = Motion Profile, F = Percent Output"=FALSE) -> (w445:T25)
      }
      frame "Finish" {
        n71 = disable-structure shown="Enabled" {
          disable-tunnel: w462 -> [w464 w468]
          disable-tunnel: [w463 w467] -> w460
          frame Disabled {
            n72 = Bundle By Name(cluster=w464, "Joystick VS Vision Latch"=FALSE) -> (w463:T25)
          }
          frame Enabled {
            n73 = Bundle By Name(cluster=w468, "Vision States"=Vision_States."Ready") -> (w467:T25)
          }
        }
        n74 = Bundle By Name(cluster=w460, "Start Motion Profile?"=FALSE ("T = Motion Profile, F = Percent Output")) -> (w458:T25)
        n75 = Bundle By Name(cluster=w458, "T = Motion Profile, F = Percent Output"=FALSE) -> (w457:T25)
      }
      frame "Test Disabled" {
        n76 = disable-structure shown="Enabled" {
          disable-tunnel: w474 -> [w476 w480]
          disable-tunnel: [w475 w479] -> w472
          frame Disabled {
            n77 = Bundle By Name(cluster=w476, "Joystick VS Vision Latch"=FALSE) -> (w475:T25)
          }
          frame Enabled {
            n78 = Bundle By Name(cluster=w480, "Vision States"=Vision_States."Ready") -> (w479:T25)
          }
        }
        n79 = Bundle By Name(cluster=w472, "Start Motion Profile?"=FALSE ("T = Motion Profile, F = Percent Output")) -> (w470:T25)
        n80 = Bundle By Name(cluster=w470, "T = Motion Profile, F = Percent Output"=FALSE) -> (w469:T25)
      }
      frame "Test Enabled" {
        n81 = Bundle By Name(cluster=w494, "DriveJoystickDevRef"=w493, "Drive Axes"=w492, "Drive Buttons"=w491, "Drive POVs"=w490, "AuxJoystickDevRef"=w489, "Aux Axes"=w488, "Aux Buttons"=w487, "Aux POVs"=w486) -> (w484:T25)
        n82 = Bundle By Name(cluster=w484, "Start Motion Profile?"=FALSE ("T = Motion Profile, F = Percent Output")) -> (w482:T25)
        n83 = Bundle By Name(cluster=w482, "T = Motion Profile, F = Percent Output"=FALSE) -> (w481:T25)
      }
      frame "Emergency Stopped" {
        n84 = disable-structure shown="Enabled" {
          disable-tunnel: w500 -> [w502 w506]
          disable-tunnel: [w501 w505] -> w498
          frame Disabled {
            n85 = Bundle By Name(cluster=w502, "Joystick VS Vision Latch"=FALSE) -> (w501:T25)
          }
          frame Enabled {
            n86 = Bundle By Name(cluster=w506, "Vision States"=Vision_States."Ready") -> (w505:T25)
          }
        }
        n87 = Bundle By Name(cluster=w498, "Start Motion Profile?"=FALSE ("T = Motion Profile, F = Percent Output")) -> (w496:T25)
        n88 = Bundle By Name(cluster=w496, "T = Motion Profile, F = Percent Output"=FALSE) -> (w495:T25)
      }
    }
    n89 = Wait (ms)(milliseconds to wait=u32 50) -> ()  [unwired: 1 out]
    n90 = call-poly <vilib>:"NT Write Value.vi"("Numeric"=1, "Name"="/limelight/stream") -> ()  [unwired: 9 in, 1 out]
    n91 = Unbundle By Name(w171) -> ("Drive Motors.Motors[]"=w170:T1[])
    n92 = Unbundle By Name(w171) -> ("Drive Buttons"=w177:bool[])
    n93 = Unbundle By Name(w171) -> ("Drive Button Indexes.A Button"=w194:i32)
    n94 = Unbundle By Name(w171) -> ("Drive Axes Indexes.Left X"=w179:i32, "Drive Axes Indexes.Left Y"=w180:i32, "Drive Axes Indexes.Right X"=w181:i32, "Drive Axes Indexes.Right Y"=w182:i32)
    n95 = Unbundle By Name(w171) -> ("Drive Buttons"=w176:bool[])
    n96 = Unbundle By Name(w171) -> ("Drive Button Indexes.LB Button"=w175:i32)
    n97 = Unbundle By Name(w171) -> ("Joystick VS Vision Latch"=w196:bool)
    n98 = Unbundle By Name(w171) -> ("Drive Axes"=w178:dbl[])
    n99 = global read "Robot Global Data.vi" "Robot Mode"() -> (w183:T17)
    n100 = Index Array(array=w170, index #1=2 ("index"), index #2=3 ("index")) -> (element #1=w169:T1, element #2=w168:T1)
    n101 = Bundle By Name(cluster=w171, "Robot Mode"=w183) -> (w197:T25)
    n102 = Index Array(array=w177, index=w194) -> (element=w195:bool)
    n103 = global read "Robot Global Data.vi" "Which Robot?"() -> (w141:T29)
    n104 = Index Array(array=w178, index #1=w179, index #2=w180, index #3=w181, index #4=w182) -> (element #1=w187:dbl, element #2=w188:dbl, element #3=w189:dbl, element #4=w190:dbl)
    n105 = global read "Robot Global Data.vi" "Which Robot?"() -> (w147:T29)
    n106 = Index Array(array=w176, index=w175) -> (element=w173:bool)
    n107 = global read "Robot Global Data.vi" "Right Encoder Val. Initial"() -> (w148:dbl)
    n108 = global read "Robot Global Data.vi" "Left Encoder Val. Initial"() -> (w150:dbl)
    n109 = disable-structure shown="Enabled" {
      disable-tunnel: w195 -> [w382 w389]
      disable-tunnel: w196 -> [_ w387]
      disable-tunnel: w197 -> [_ w385]
      disable-tunnel: [_ w383] -> w174
      frame Disabled {
        n110 = feedback #2() -> (w381:bool)  [unwired: 1 in]
        n111 = feedback-in #2(w382) -> ()
        n112 = Greater?(x=w382, y=w381) -> (0:w380:bool)
        n113 = global write "Robot Global Data.vi" "Driver VS Vision Control"(w380) -> ()
      }
      frame Enabled {
        n114 = feedback #3() -> (w390:bool)  [unwired: 1 in]
        n115 = feedback-in #3(w389) -> ()
        n116 = Greater?(x=w389, y=w390) -> (0:w388:bool)
        n117 = Not(x=w387) -> (.not. x?=w386:bool)
        n118 = Select(t=w386, s=w388, f=w387) -> (s? t:f=w384:bool)
        n119 = global write "Robot Global Data.vi" "Driver VS Vision Control"(w384) -> ()
        n120 = Bundle By Name(cluster=w385, "Joystick VS Vision Latch"=w384) -> (w383:T25)
      }
    }
    n121 = call "Deadband.vi"("Input"=w187) -> ("Output"=w185:dbl)  [unwired: 10 in]
    n122 = call "Deadband.vi"("Input"=w188) -> ("Output"=w186:dbl)  [unwired: 10 in]
    n123 = call "Deadband.vi"("Input"=w189) -> ("Output"=w184:dbl)  [unwired: 10 in]
    n124 = call "Deadband.vi"("Input"=w190) -> ("Output"=w191:dbl)  [unwired: 10 in]
    n125 = call-poly <vilib>:"CTRE_Phoenix_MotorController_Get_Enhanced.vi"("PhoenixMotorControlDevRef"=w169) -> ("Quadrature Position"=w151:i32)  [unwired: 11 in, 3 out]
    n126 = call-poly <vilib>:"CTRE_Phoenix_MotorController_Get_Enhanced.vi"("PhoenixMotorControlDevRef"=w168) -> ("Quadrature Position"=w149:i32)  [unwired: 11 in, 3 out]
    n127 = Negate(x=w186) -> (-x=w192:dbl)
    n128 = Negate(x=w191) -> (-x=w193:dbl)
    n129 = global write "Robot Global Data.vi" "Left Drive Joystick X"(w185) -> ()
    n130 = global write "Robot Global Data.vi" "Right Drive Joystick X"(w184) -> ()
    n131 = case shown="\"Competition Bot\", Default" w141 {
      tunnel: [w213 w215 w217] -> w140
      tunnel: [w212 w214 w216] -> w139
      frame "Competition Bot", Default {
        w212 = 18069  # Change in Encoder
        w213 = 84  # Change in Distance (inches)
      }
      frame "Practice Bot" {
        w214 = 0  # Change in Encoder
        w215 = 0  # Change in Distance (inches)
      }
      frame "Code Bot" {
        w216 = 0  # Change in Encoder
        w217 = 0  # Change in Distance (inches)
      }
    }
    n132 = global write "Robot Global Data.vi" "Right Drive Joystick Y"(w193) -> ()
    n133 = global write "Robot Global Data.vi" "Left Drive Joystick Y"(w192) -> ()
    n134 = case shown="\"Competition Bot\", Default" w147 {
      tunnel: [w219 w221 w223] -> w146
      tunnel: [w218 w220 w222] -> w145
      frame "Competition Bot", Default {
        w218 = 17996  # Change in Encoder
        w219 = 84  # Change in Distance (inches)
      }
      frame "Practice Bot" {
        w220 = 0  # Change in Encoder
        w221 = 0  # Change in Distance (inches)
      }
      frame "Code Bot" {
        w222 = 0  # Change in Encoder
        w223 = 0  # Change in Distance (inches)
      }
    }
    n135 = Subtract(x=w151, y=w150) -> (x-y=w143:dbl)
    n136 = Subtract(x=w149, y=w148) -> (x-y=w137:dbl)
    n137 = Bundle By Name(cluster=w174, "Vision Track Mode Override"=w173) -> (w126:T25)
    n138 = global write "Robot Global Data.vi" "Right Encoder in Enc. Vals"(w137) -> ()
    n139 = global write "Robot Global Data.vi" "Left Encoder in Enc. Vals"(w143) -> ()
    n140 = Divide(x=w140, y=w139) -> (x/y=w136:dbl)
    n141 = Divide(x=w146, y=w145) -> (x/y=w144:dbl)
    n142 = Multiply(x=w144, y=w143) -> (x*y=w142:dbl)
    n143 = Multiply(x=w137, y=w136) -> (x*y=w138:dbl)
    n144 = global write "Robot Global Data.vi" "Left Encoder in Inches"(w142) -> ()
    n145 = global write "Robot Global Data.vi" "Right Encoder in Inches"(w138) -> ()
    n146 = disable-structure shown="Enabled" {
      disable-tunnel: w126 -> [w273 w280]
      frame Disabled {
        n147 = Unbundle By Name(w273) -> ("Drive Button Indexes.RB Button"=w272:i32)
        n148 = Unbundle By Name(w273) -> ("Drive Buttons"=w271:bool[])
        n149 = Unbundle By Name(w273) -> ("T = Motion Profile, F = Percent Output"=w266:bool)
        n150 = Index Array(array=w271, index=w272) -> (element=w269:bool)
        n151 = feedback #4() -> (w270:bool)  [unwired: 1 in]
        n152 = feedback-in #4(w269) -> ()
        n153 = Greater?(x=w269, y=w270) -> (0:w268:bool)
        n154 = Not(x=w266) -> (.not. x?=w267:bool)
        n155 = Select(t=w267, s=w268, f=w266) -> ()  [unwired: 1 out]
      }
      frame Enabled {
        n156 = Unbundle By Name(w280) -> ("Drive Button Indexes.Y Button"=w282:i32)
        n157 = Unbundle By Name(w280) -> ("Drive Buttons"=w281:bool[])
        n158 = global read "Robot Global Data.vi" "Cancel the Motion Profile?"() -> (w274:bool)
        n159 = Index Array(array=w281, index=w282) -> (element=w276:bool)
        n160 = feedback #5() -> (w279:bool)  [unwired: 1 in]
        n161 = feedback-in #5(w276) -> ()
        n162 = Greater?(x=w276, y=w279) -> (0:w278:bool)
        n163 = Not(x=w274) -> (.not. x?=w277:bool)
        n164 = Select(t=w277, s=w278, f=w274) -> (s? t:f=w275:bool)
        n165 = global write "Robot Global Data.vi" "Cancel the Motion Profile?"(w275) -> ()
      }
    }
    n166 = Unbundle By Name(w126) -> ("Drive Button Indexes.RB Button"=w133:i32)
    n167 = Unbundle By Name(w126) -> ("Drive Buttons"=w132:bool[])
    n168 = Index Array(array=w132, index=w133) -> (element=w131:bool)
    n169 = Bundle By Name(cluster=w126, "Arcade Drive?"=w131) -> (w125:T25)
    n170 = call "RIGHT Motion Profile Traj Points Array.vi"("Read = false, Write = true"=FALSE) -> ("traj. points array out"=w152:dbl[][])  [unwired: 10 in]
    "Right Traj. Pts Array" <- w152
    n171 = call "LEFT Motion Profile Traj Points Array.vi"("Read = false, Write = true"=FALSE) -> ("traj. points array out"=w159:dbl[][])  [unwired: 10 in]
    "Left Traj. Pts Array" <- w159
    n172 = for {
      N -> [w237]
      tunnel: w152 -> [w243] mode=indexing
      tunnel: [w233] -> w158 mode=indexing
      i -> [w236]
      w242 = 0.0 ("Arbitrary Feed Forward")
      # "Convert profile units to talon units"
      n173 = Decrement(x=w237) -> (x-1=w238:i32)
      n174 = Equal?(x=w238, y=w236) -> (x = y?=w239:bool)
      n175 = Equal To 0?(x=w236) -> (x = 0?=w235:bool)
      n176 = Index Array(array=w243) -> (element #1=w231:dbl, element #2=w225:dbl, element #3=w232:dbl)  [unwired: 3 in]
      n177 = Multiply(x=4096.0, y=w225) -> (x*y=w227:dbl)
      n178 = Multiply(x=4096.0, y=w231) -> (x*y=w229:dbl)
      n179 = Divide(x=w227, y=10.0) -> (x/y=w224:dbl)
      n180 = Bundle By Name(cluster=T28 {"Position"=0.0, "Velocity"=0.0, "Arbitrary Feed Forward"=0.0, "Auxiliary Position"=0.0, "Auxiliary Velocity"=0.0, "Auxiliary Arbitrary Feed Forward"=0.0, "Profile Slot Select"=0, "Auxiliary Profile Slot Select"=0, "isLastPoint?"=FALSE, "Zero Position?"=FALSE, "durationMs"=0, "Use Aux PID?"=FALSE} ("Trajectory Point"), "Position"=w229, "Velocity"=w224, "Arbitrary Feed Forward"=w242, "Auxiliary Position"=w242, "Auxiliary Velocity"=w242, "Auxiliary Arbitrary Feed Forward"=w242, "Profile Slot Select"=0, "Auxiliary Profile Slot Select"=1, "isLastPoint?"=w239, "Zero Position?"=w235, "durationMs"=w232, "Use Aux PID?"=FALSE) -> (w233:T28)
    }
    n181 = for {
      N -> [w258]
      tunnel: w159 -> [w264] mode=indexing
      tunnel: [w254] -> w165 mode=indexing
      i -> [w257]
      w263 = 0.0 ("Arbitrary Feed Forward")
      # "Convert profile units to talon units"
      n182 = Decrement(x=w258) -> (x-1=w259:i32)
      n183 = Equal?(x=w259, y=w257) -> (x = y?=w260:bool)
      n184 = Equal To 0?(x=w257) -> (x = 0?=w256:bool)
      n185 = Index Array(array=w264) -> (element #1=w252:dbl, element #2=w246:dbl, element #3=w253:dbl)  [unwired: 3 in]
      n186 = Multiply(x=4096.0, y=w246) -> (x*y=w248:dbl)
      n187 = Multiply(x=4096.0, y=w252) -> (x*y=w250:dbl)
      n188 = Divide(x=w248, y=10.0) -> (x/y=w245:dbl)
      n189 = Bundle By Name(cluster=T28 {"Position"=0.0, "Velocity"=0.0, "Arbitrary Feed Forward"=0.0, "Auxiliary Position"=0.0, "Auxiliary Velocity"=0.0, "Auxiliary Arbitrary Feed Forward"=0.0, "Profile Slot Select"=0, "Auxiliary Profile Slot Select"=0, "isLastPoint?"=FALSE, "Zero Position?"=FALSE, "durationMs"=0, "Use Aux PID?"=FALSE} ("Trajectory Point"), "Position"=w250, "Velocity"=w245, "Arbitrary Feed Forward"=w263, "Auxiliary Position"=w263, "Auxiliary Velocity"=w263, "Auxiliary Arbitrary Feed Forward"=w263, "Profile Slot Select"=0, "Auxiliary Profile Slot Select"=1, "isLastPoint?"=w260, "Zero Position?"=w256, "durationMs"=w253, "Use Aux PID?"=FALSE) -> (w254:T28)
    }
    n190 = call <vilib>:"CTRE_Phoenix_MotorControl_BufferedTrajectoryPointStream_Open.vi"() -> ("BufferedTrajectoryPointStream_DevRef"=w157:T30)  [unwired: 10 in, 1 out]
    n191 = call <vilib>:"CTRE_Phoenix_MotorControl_BufferedTrajectoryPointStream_Open.vi"() -> ("BufferedTrajectoryPointStream_DevRef"=w164:T30)  [unwired: 10 in, 1 out]
    n192 = call-poly <vilib>:"CTRE_Phoenix_MotorControl_BufferedTrajectoryPointStream_Write.vi"("Motion Profile Trajectory Point Array"=w158, "BufferedTrajectoryPointStream_DevRef"=w157) -> ("error out"=w155:errorcluster, "BufferedTrajectoryPointStream_DevRef"=w156:T30)  [unwired: 8 in]
    n193 = call-poly <vilib>:"CTRE_Phoenix_MotorControl_BufferedTrajectoryPointStream_Write.vi"("Motion Profile Trajectory Point Array"=w165, "BufferedTrajectoryPointStream_DevRef"=w164) -> ("error out"=w162:errorcluster, "BufferedTrajectoryPointStream_DevRef"=w163:T30)  [unwired: 8 in]
    n194 = call <vilib>:"CTRE_Phoenix_MotorControl_BufferedTrajectoryPointStream_SetDeviceReference.vi"("error in (no error)"=w155, "refnum name"="right_mpStream", "BufferedTrajectoryPointStream_DevRef"=w156) -> ()  [unwired: 7 in, 2 out]
    n195 = call <vilib>:"CTRE_Phoenix_MotorControl_BufferedTrajectoryPointStream_SetDeviceReference.vi"("error in (no error)"=w162, "refnum name"="left_mpStream", "BufferedTrajectoryPointStream_DevRef"=w163) -> ()  [unwired: 7 in, 2 out]
    n196 = Unbundle By Name(w125) -> ("T = Motion Profile, F = Percent Output"=w130:bool)
    n197 = Unbundle By Name(w125) -> ("Start Motion Profile?"=w124:bool)
    n198 = case shown="False" w130 {
      tunnel: [w284 w376] -> w210
      tunnel: w125 -> [w283 w377]
      tunnel: w124 -> [_ w375]
      frame False {
        n199 = disable-structure shown="Enabled" {
          disable-tunnel: [w300 w320] -> w284
          disable-tunnel: w283 -> [w292 w306]
          frame Enabled {
            # "Vision and Joystick Control for Drive Train"
            # "for ease of testing\nfor programmers"
            # "1 = force off\n3 = force on"
            # "0 = vision processor\n1 = driver camera settings"
            n200 = Unbundle By Name(w292) -> ("Joystick VS Vision Latch"=w296:bool)
            n201 = Unbundle By Name(w292) -> ("Vision Track Mode Override"=w288:bool)
            n202 = Select(t=3, s=w296, f=1) -> (s? t:f=w287:i32)
            n203 = Select(t=0, s=w296, f=1) -> (s? t:f=w291:i32)
            n204 = Select(t=3, s=w288, f=w287) -> (s? t:f=w286:i32)
            n205 = Select(t=0, s=w288, f=w291) -> (s? t:f=w289:i32)
            n206 = case shown="True" w296 {
              tunnel: w292 -> [w301 w303]
              tunnel: [w301 w304] -> w300
              frame False {
                n207 = Unbundle By Name(w301) -> ("Arcade Drive?"=w302:bool)
                n208 = call "Joystick Drive Control.vi"("Arcade Drive?"=w302, "Cluster In"=w301) -> ()  [unwired: 10 in]
              }
              frame True {
                n209 = call "Vision Tracking Drive Control.vi"("Cluster In"=w303) -> ("Cluster Out"=w304:T25)  [unwired: 10 in]
              }
            }
            n210 = call-poly <vilib>:"NT Write Value.vi"("Numeric"=w289, "Name"="/limelight/camMode") -> ()  [unwired: 9 in, 1 out]
            n211 = call-poly <vilib>:"NT Write Value.vi"("Numeric"=w286, "Name"="/limelight/ledMode") -> ()  [unwired: 9 in, 1 out]
          }
          frame Disabled {
            n212 = call-poly <vilib>:"NT Read Value.vi"("Name"="/limelight/tx") -> ("Numeric"=w314:dbl)  [unwired: 9 in, 1 out]
            n213 = call-poly <vilib>:"NT Read Value.vi"("Name"="/limelight/ty") -> ("Numeric"=w313:dbl)  [unwired: 9 in, 1 out]
            n214 = call-poly <vilib>:"NT Read Value.vi"("Name"="/limelight/ta") -> ("Numeric"=w312:dbl)  [unwired: 9 in, 1 out]
            n215 = call-poly <vilib>:"NT Read Value.vi"("Name"="/limelight/ts") -> ("Numeric"=w311:dbl)  [unwired: 9 in, 1 out]
            n216 = call-poly <vilib>:"NT Read Value.vi"("Name"="/limelight/tshort") -> ("Numeric"=w308:dbl)  [unwired: 9 in, 1 out]
            n217 = call-poly <vilib>:"NT Read Value.vi"("Name"="/limelight/tlong") -> ("Numeric"=w307:dbl)  [unwired: 9 in, 1 out]
            n218 = Bundle By Name(cluster=w306, "limelight.offsetAngle H"=w314, "limelight.offsetAngle V"=w313, "limelight.area"=w312, "limelight.skew"=w311, "limelight.shortest side (pxls)"=w308, "limelight.longest side (pxls)"=w307) -> (w305:T25)
            n219 = Unbundle By Name(w305) -> ("Vision States"=w322:T19)
            n220 = case shown="\"Ready\", Default" w322 {
              tunnel: [w323 w338 w356] -> w321
              tunnel: w305 -> [w323 w338 w356]
              tunnel: [w332 w339 w352] -> w319
              frame "Ready", Default {
                # "should have created a \nboolean in the cluster \ninstead of just pulling\nthe A button"
                # "the Ys of the drive joysticks are \ninverted by default"
                n221 = Unbundle By Name(w323) -> ("Drive Button Indexes.A Button"=w337:i32)
                n222 = Unbundle By Name(w323) -> ("Drive Buttons"=w336:bool[])
                n223 = Unbundle By Name(w323) -> ("Drive Motors"=w331:T11, "Drive Axes"=w330:dbl[], "Drive Axes Indexes.Left Y"=w329:i32, "Drive Axes Indexes.Right Y"=w328:i32)
                n224 = Index Array(array=w336, index=w337) -> (element=w335:bool)
                n225 = Index Array(array=w330, index #1=w329, index #2=w328) -> (element #1=w327:dbl, element #2=w326:dbl)
                n226 = Negate(x=w327) -> (-x=w324:dbl)
                n227 = Negate(x=w326) -> (-x=w325:dbl)
                n228 = Select(t=Vision_States."Forward Until Target at Edge" ("Vision States"), s=w335, f=Vision_States."Ready" ("Vision States")) -> (s? t:f=w332:T19)
                n229 = call <vilib>:"WPI_RobotDriveTankDrive.vi"("Right axis value"=w325, "Left axis value"=w324, "RobotDriveDevRef"=w331) -> ()  [unwired: 6 in, 3 out]
              }
              frame "Forward Until Target at Edge" {
                n230 = Unbundle By Name(w338) -> ("limelight.offsetAngle H"=w343:dbl)
                n231 = Less?(x=w343, y=-26) -> (x < y?=w341:bool)
                n232 = Greater?(x=w343, y=14) -> (0:w342:bool)
                n233 = Or(x=w342, y=w341) -> (x .or. y?=w340:bool)
                n234 = case shown="False" w340 {
                  tunnel: [Vision_States."Forward Until Target at Edge" ("Vision States") Vision_States."Vision Track" ("Vision States")] -> w339
                  tunnel: w338 -> [w349 _]
                  frame False {
                    w347 = 0.35
                    n235 = Unbundle By Name(w349) -> ("Drive Motors"=w348:T11)
                    n236 = call <vilib>:"WPI_RobotDriveTankDrive.vi"("Right axis value"=w347, "Left axis value"=w347, "RobotDriveDevRef"=w348) -> ()  [unwired: 6 in, 3 out]
                  }
                  frame True {
                  }
                }
              }
              frame "Vision Track" {
                w359 = 0.5 ("t")
                w358 = 1.5
                # "this is the target area for\nwhen to stop driving \ntoward target (10 here \nwould means 10% of \nlimelight feed)"
                # "Hori. offset scaled down to\nbe a reasonable drive speed\ncoefficient (e.g. if this number\nis 0.01, 10deg offset to the \nleft would make right train \nrun at 110% and left train \nat 90%)"
                # "0deg offset = speed \nadjustment coefficient of 1"
                n237 = Unbundle By Name(w356) -> ("limelight.area"=w364:dbl, "limelight.offsetAngle H"=w372:dbl)
                n238 = Multiply(x=w372, y=0.03) -> (x*y=w361:dbl)
                n239 = Unbundle By Name(w356) -> ("Drive Motors"=w357:T11)
                n240 = Add(x=1.0, y=w361) -> (x+y=w367:dbl)
                n241 = Subtract(x=1.0, y=w361) -> (x-y=w360:dbl)
                n242 = Less?(x=w364, y=w358) -> (x < y?=w355:bool)
                n243 = Less?(x=w364, y=w358) -> (x < y?=w368:bool)
                n244 = Select(t=w359, s=w355, f=0.0) -> (s? t:f=w373:dbl)
                n245 = Select(t=w359, s=w368, f=0.0) -> (s? t:f=w365:dbl)
                n246 = Multiply(x=w373, y=w367) -> (x*y=w370:dbl)
                n247 = Multiply(x=w360, y=w365) -> (x*y=w363:dbl)
                n248 = Not(x=w355) -> (.not. x?=w351:bool)
                n249 = call <vilib>:"WPI_RobotDriveTankDrive.vi"("Right axis value"=w363, "Left axis value"=w370, "RobotDriveDevRef"=w357) -> ()  [unwired: 6 in, 3 out]
                n250 = Select(t=Vision_States."Ready" ("Vision States"), s=w351, f=Vision_States."Vision Track" ("Vision States")) -> (s? t:f=w352:T19)
              }
            }
            n251 = Bundle By Name(cluster=w321, "Vision States"=w319) -> (w320:T25)
          }
        }
      }
      frame True {
        # "left MP will control when the motion profile ends"
        # "Motion Profile Control for Drive Train"
        n252 = call "Motion Profile Left Drive Control.vi"("Start Motion Profile?"=w375, "Cluster In"=w377) -> ("Cluster Out"=w376:T25)  [unwired: 9 in]
        n253 = call "Motion Profile Right Drive Control.vi"("Start Motion Profile?"=w375, "Cluster In"=w377) -> ()  [unwired: 9 in, 1 out]
      }
    }
  }
  n254 = while {
    shift-right: [w510] -> _
    shift-left: w84 -> [w556]
    stop <- FALSE stop-if-true
    # "this chunk of code \ncontrols the wanted\nangle of the collector\nusing a joystick and\n2 angle presets"
    # "use this to scale the rate at which the\nwanted angle changes based on the joystick"
    # "we use this to set the\n\"0\" of the encoder to be \nwherever it is when the code\nis run (or the robot is turned\non in the case of \nhard-deployed code)"
    # "this chunk of code \nconverts the encoder\n values into angles"
    n255 = Unbundle By Name(w556) -> ("DriveJoystickDevRef"=w567:T9)
    n256 = Unbundle By Name(w556) -> ("AuxJoystickDevRef"=w566:T9)
    n257 = Unbundle By Name(w556) -> ("Robot Mode"=w565:T17)
    n258 = Wait (ms)(milliseconds to wait=u32 50) -> ()  [unwired: 1 out]
    n259 = call <vilib>:"WPI_JoystickGetValues.vi"("JoystickDevRef"=w566) -> ("Buttons"=w558:bool[], "Axes"=w559:dbl[], "JoystickDevRef"=w560:T9, "POVs"=w557:i16[])  [unwired: 6 in, 1 out]
    n260 = call <vilib>:"WPI_JoystickGetValues.vi"("JoystickDevRef"=w567) -> ("Buttons"=w562:bool[], "Axes"=w564:dbl[], "JoystickDevRef"=w563:T9, "POVs"=w561:i16[])  [unwired: 6 in, 1 out]
    n261 = case shown="\"Teleop Enabled\"" w565 {
      tunnel: w556 -> [w785 w795 w796 w797 w807 w808 w809 w819 w820]
      tunnel: [w785 w786 w796 w798 w807 w808 w809 w810 w820] -> w533
      tunnel: w564 -> [_ w794 _ w805 _ _ _ w817 _]
      tunnel: w563 -> [_ w793 _ w806 _ _ _ w818 _]
      tunnel: w562 -> [_ w792 _ w804 _ _ _ w816 _]
      tunnel: w561 -> [_ w791 _ w803 _ _ _ w815 _]
      tunnel: w560 -> [_ w790 _ w802 _ _ _ w814 _]
      tunnel: w559 -> [_ w789 _ w801 _ _ _ w813 _]
      tunnel: w558 -> [_ w788 _ w800 _ _ _ w812 _]
      tunnel: w557 -> [_ w787 _ w799 _ _ _ w811 _]
      frame "Autonomous Disabled", Default {
      }
      frame "Autonomous Enabled" {
        n262 = Bundle By Name(cluster=w795, "DriveJoystickDevRef"=w793, "Drive Axes"=w794, "Drive Buttons"=w792, "Drive POVs"=w791, "AuxJoystickDevRef"=w790, "Aux Axes"=w789, "Aux Buttons"=w788, "Aux POVs"=w787) -> (w786:T26)
      }
      frame "Teleop Disabled" {
      }
      frame "Teleop Enabled" {
        n263 = Bundle By Name(cluster=w797, "DriveJoystickDevRef"=w806, "Drive Axes"=w805, "Drive Buttons"=w804, "Drive POVs"=w803, "AuxJoystickDevRef"=w802, "Aux Axes"=w801, "Aux Buttons"=w800, "Aux POVs"=w799) -> (w798:T26)
      }
      frame "Disconnected" {
      }
      frame "Finish" {
      }
      frame "Test Disabled" {
      }
      frame "Test Enabled" {
        n264 = Bundle By Name(cluster=w819, "DriveJoystickDevRef"=w818, "Drive Axes"=w817, "Drive Buttons"=w816, "Drive POVs"=w815, "AuxJoystickDevRef"=w814, "Aux Axes"=w813, "Aux Buttons"=w812, "Aux POVs"=w811) -> (w810:T26)
      }
      frame "Emergency Stopped" {
      }
    }
    n265 = Unbundle By Name(w533) -> ("Aux Button Indexes.RB Button"=w531:i32)
    n266 = Unbundle By Name(w533) -> ("Aux Button Indexes.RT Button"=w530:i32)
    n267 = Unbundle By Name(w533) -> ("Aux Joystick Indexes.Right Y"=w540:i32)
    n268 = Unbundle By Name(w533) -> ("Aux Button Indexes.LT Button"=w554:i32)
    n269 = Unbundle By Name(w533) -> ("Aux Axes"=w541:dbl[])
    n270 = Unbundle By Name(w533) -> ("Aux Buttons"=w532:bool[])
    n271 = Unbundle By Name(w533) -> ("Aux Buttons"=w553:bool[])
    n272 = Unbundle By Name(w533) -> ("Hatch Collector Wanted Angle"=w538:dbl)
    n273 = Unbundle By Name(w533) -> ("Hatch Retainer Move Up/Down"=w550:bool)
    n274 = Unbundle By Name(w533) -> ("HatchCollectorMotorDevRef"=w547:T1)
    n275 = global read "Robot Global Data.vi" "Hatch Encoder Start Value"() -> (w542:dbl)
    n276 = global read "Robot Global Data.vi" "Robot Mode"() -> (w555:T17)
    n277 = global read "Robot Global Data.vi" "Which Robot?"() -> (w518:T29)
    n278 = Bundle By Name(cluster=w533, "Robot Mode"=w555) -> (w552:T26)
    n279 = call-poly <vilib>:"CTRE_Phoenix_MotorController_Get_Enhanced.vi"("PhoenixMotorControlDevRef"=w547) -> ("Quadrature Position"=w545:i32)  [unwired: 11 in, 3 out]
    n280 = Index Array(array=w541, index=w540) -> (element=w524:dbl)
    n281 = Index Array(array=w553, index=w554) -> (element=w551:bool)
    n282 = Index Array(array=w532, index #1=w531, index #2=w530) -> (element #1=w527:bool, element #2=w528:bool)
    n283 = call "Deadband.vi"("Input"=w524) -> ("Output"=w522:dbl)  [unwired: 10 in]
    n284 = disable-structure shown="Enabled" {
      disable-tunnel: w551 -> [w740 w744]
      disable-tunnel: w550 -> [w737 _]
      disable-tunnel: [w736 w743] -> w549
      frame Disabled {
        n285 = feedback #6() -> (w741:bool)  [unwired: 1 in]
        n286 = feedback-in #6(w740) -> ()
        n287 = Greater?(x=w740, y=w741) -> (0:w739:bool)
        n288 = Not(x=w737) -> (.not. x?=w738:bool)
        n289 = Select(t=w738, s=w739, f=w737) -> (s? t:f=w736:bool)
      }
      frame Enabled {
        n290 = feedback #7() -> (w742:bool)  [unwired: 1 in]
        n291 = feedback-in #7(w744) -> ()
        n292 = Greater?(x=w744, y=w742) -> (0:w743:bool)
      }
    }
    n293 = case shown="\"Competition Bot\", Default" w518 {
      tunnel: [w760 w769 w778] -> w546
      tunnel: w545 -> [w758 w768 w777]
      tunnel: w542 -> [w759 w767 w776]
      frame "Competition Bot", Default {
        # "range of \ndegrees"
        # "enc. val at\n\"max out\"\ndeg IRL"
        # "enc. val at\n\"max in\"\ndeg IRL"
        n294 = Subtract(x=w758, y=w759) -> (x-y=w761:dbl)
        n295 = Subtract(x=1047.0, y=46.0) -> (x-y=w765:dbl)
        n296 = Divide(x=97.0, y=w765) -> (x/y=w763:dbl)
        n297 = Multiply(x=w763, y=w761) -> (x*y=w760:dbl)
      }
      frame "Practice Bot" {
        # "range of \ndegrees"
        # "enc. val at\n\"max out\"\ndeg IRL"
        # "enc. val at\n\"max in\"\ndeg IRL"
        n298 = Subtract(x=w768, y=w767) -> (x-y=w770:dbl)
        n299 = Subtract(x=1050.0, y=34.0) -> (x-y=w774:dbl)
        n300 = Divide(x=90.0, y=w774) -> (x/y=w772:dbl)
        n301 = Multiply(x=w772, y=w770) -> (x*y=w769:dbl)
      }
      frame "Code Bot" {
        # "range of \ndegrees"
        # "enc. val at\n\"max out\"\ndeg IRL"
        # "enc. val at\n\"max in\"\ndeg IRL"
        n302 = Subtract(x=w777, y=w776) -> (x-y=w779:dbl)
        n303 = Subtract(x=1050.0, y=34.0) -> (x-y=w783:dbl)
        n304 = Divide(x=90.0, y=w783) -> (x/y=w781:dbl)
        n305 = Multiply(x=w781, y=w779) -> (x*y=w778:dbl)
      }
    }
    n306 = Add(x=w538, y=w522) -> (x+y=w537:dbl)
    n307 = Or(x=w527, y=w528) -> (x .or. y?=w529:bool)
    n308 = Multiply(x=1.0, y=w537) -> (x*y=w534:dbl)
    n309 = case shown="True" w529 {
      tunnel: [w753 w754] -> w535
      tunnel: w534 -> [w753 _]
      tunnel: w527 -> [_ w755]
      frame False {
        # "neither \npreset,\nJS controls\nwanted angle"
      }
      frame True {
        n310 = case shown="True" w755 {
          tunnel: [80.0 7.0] -> w754
          frame False {
            # "preset \nfor \nhovering\nto use \ndustpan"
          }
          frame True {
            # "preset\nfor \nvertical"
          }
        }
      }
    }
    n311 = global read "Robot Global Data.vi" "Which Robot?"() -> (w517:T29)
    n312 = case shown="\"Competition Bot\", Default" w517 {
      tunnel: [97.0 99.0 90.0] -> w516
      frame "Competition Bot", Default {
        # "max deg"
      }
      frame "Practice Bot" {
        # "max deg"
      }
      frame "Code Bot" {
        # "max deg"
      }
    }
    n313 = In Range and Coerce(upper limit=w516, x=w535, lower limit=0.0) -> (coerced(x)=w526:dbl)  [unwired: 1 out]
    n314 = Bundle By Name(cluster=w552, "Hatch Retainer Move Up/Down"=w549) -> (w548:T26)
    n315 = Bundle By Name(cluster=w548, "Hatch Collector Actual Angle"=w546) -> (w539:T26)
    n316 = Bundle By Name(cluster=w539, "Hatch Collector Wanted Angle"=w526) -> (w511:T26)
    n317 = disable-structure shown="Enabled" {
      disable-tunnel: [w660 w683] -> w512
      disable-tunnel: w511 -> [w658 w693]
      disable-tunnel: w511 -> [w657 w686]
      frame Disabled {
        # "only let kickers kick\nif the hatch retainer\nis fully down"
        # "if kick button was just pressed, go\ndown. Otherwise, keep the states\nas they are"
        n318 = Unbundle By Name(w657) -> ("KickerSolenoidDevRef"=w675:T6)
        n319 = Unbundle By Name(w657) -> ("Hatch Retainer States"=w662:T14)
        n320 = Unbundle By Name(w657) -> ("Aux Button Indexes.LB Button"=w673:i32)
        n321 = Unbundle By Name(w657) -> ("Aux Buttons"=w674:bool[])
        n322 = global read "Robot Global Data.vi" "Kick Hatch in Auto"() -> (w668:bool)
        n323 = case shown="\"Fully Down (not retained)\", Default" w662 {
          tunnel: [TRUE FALSE FALSE FALSE] -> w666
          frame "Fully Down (not retained)", Default {
          }
          frame "Going Up" {
          }
          frame "Fully Up (retained)" {
          }
          frame "Going Down" {
          }
        }
        n324 = Index Array(array=w674, index=w673) -> (element=w669:bool)
        n325 = Or(x=w669, y=w668) -> (x .or. y?=w664:bool)
        n326 = And(x=w664, y=w666) -> (x .and. y?=w667:bool)
        n327 = feedback #8() -> (w665:bool)  [unwired: 1 in]
        n328 = feedback-in #8(w664) -> ()
        n329 = Select(t=WPI_SolenoidValue."On" ("Value"), s=w667, f=WPI_SolenoidValue."Off" ("Value")) -> (s? t:f=w670:T31)
        n330 = Greater?(x=w664, y=w665) -> (0:w663:bool)
        n331 = call-poly <vilib>:"WPI_SolenoidSet.vi"("Value"=w670, "SolenoidDevRef"=w675) -> ()  [unwired: 8 in, 2 out]
        n332 = Select(t=Hatch_Retainer_States."Going Down" ("Hatch Retainer States"), s=w663, f=w662) -> (s? t:f=w661:T14)
        n333 = Bundle By Name(cluster=w658, "Hatch Retainer States"=w661) -> (w660:T26)
      }
      frame Enabled {
        n334 = Unbundle By Name(w686) -> ("Aux Button Indexes.LB Button"=w691:i32)
        n335 = Unbundle By Name(w686) -> ("Hatch Kicking States"=w681:T12)
        n336 = Unbundle By Name(w686) -> ("Aux Buttons"=w692:bool[])
        n337 = Unbundle By Name(w686) -> ("Hatch Retainer States"=w685:T14)
        n338 = Unbundle By Name(w686) -> ("KickerSolenoidDevRef"=w690:T6)
        n339 = feedback #9() -> (w680:T12)  [unwired: 1 in]
        n340 = feedback-in #9(w681) -> ()
        n341 = Index Array(array=w692, index=w691) -> (element=w687:bool)
        n342 = case shown="\"Kick Hatch\"" w681 {
          selector: w681 -> [_ _ w718]
          tunnel: [WPI_SolenoidValue."Off" ("Value") WPI_SolenoidValue."Off" ("Value") w715] -> w689
          tunnel: [w695 w702 w719] -> w688
          tunnel: w687 -> [w698 _ _]
          tunnel: w685 -> [w694 w700 w723]
          tunnel: [w694 w703 w723] -> w682
          tunnel: w680 -> [_ _ w716]
          frame "Ready", Default {
            n343 = Select(t=Hatch_Kicking_States."Stop Retaining Hatch" ("Hatch Kicking States"), s=w698, f=Hatch_Kicking_States."Ready" ("Hatch Kicking States")) -> (s? t:f=w695:T12)
          }
          frame "Stop Retaining Hatch" {
            n344 = Equal?(x=Hatch_Retainer_States."Fully Down (not retained)" ("Hatch Retainer States"), y=w700) -> (x = y?=w704:bool)
            n345 = case shown="False" w704 {
              tunnel: [Hatch_Retainer_States."Going Down" ("Hatch Retainer States") Hatch_Retainer_States."Fully Down (not retained)" ("Hatch Retainer States")] -> w703
              tunnel: [Hatch_Kicking_States."Stop Retaining Hatch" ("Hatch Kicking States") Hatch_Kicking_States."Kick Hatch" ("Hatch Kicking States")] -> w702
              frame False {
              }
              frame True {
              }
            }
          }
          frame "Kick Hatch" {
            # "if previous state\nis not the same \nas the current, we\njust entered \"kick\nhatch\" and \nshould reset our\ntimer"
            n346 = Not Equal?(x=w718, y=w716) -> (x != y?=w717:bool)
            n347 = call "Elapsed Time"("Reset"=w717) -> ("Elapsed Time (s)"=w713:dbl)  [unwired: 11 in, 7 out]
            n348 = Greater Or Equal?(x=w713, y=1.5) -> (x >= y?=w722:bool)
            n349 = Less Or Equal?(x=w713, y=0.5) -> (x <= y?=w714:bool)
            n350 = Select(t=WPI_SolenoidValue."On" ("Value"), s=w714, f=WPI_SolenoidValue."Off" ("Value")) -> (s? t:f=w715:T31)
            n351 = Select(t=Hatch_Kicking_States."Ready" ("Hatch Kicking States"), s=w722, f=Hatch_Kicking_States."Kick Hatch" ("Hatch Kicking States")) -> (s? t:f=w719:T12)
          }
        }
        n352 = Bundle By Name(cluster=w693, "Hatch Kicking States"=w688) -> (w684:T26)
        n353 = Bundle By Name(cluster=w684, "Hatch Retainer States"=w682) -> (w683:T26)
        n354 = call-poly <vilib>:"WPI_SolenoidSet.vi"("Value"=w689, "SolenoidDevRef"=w690) -> ()  [unwired: 8 in, 2 out]
      }
    }
    n355 = Unbundle By Name(w511) -> ("RetainerSolenoidDevRef"=w509:T6)
    n356 = disable-structure shown="Disabled" {
      disable-tunnel: w511 -> [w745 _]
      frame Disabled {
        n357 = Unbundle By Name(w745) -> ("Aux Button Indexes.B Button"=w752:i32)
        n358 = Unbundle By Name(w745) -> ("LifterSolenoidDevRef"=w746:T6)
        n359 = Unbundle By Name(w745) -> ("Aux Buttons"=w751:bool[])
        n360 = Index Array(array=w751, index=w752) -> (element=w748:bool)
        n361 = Select(t=WPI_SolenoidValue."On" ("Value"), s=w748, f=WPI_SolenoidValue."Off" ("Value")) -> (s? t:f=w747:T31)
        n362 = call-poly <vilib>:"WPI_SolenoidSet.vi"("Value"=w747, "SolenoidDevRef"=w746) -> ()  [unwired: 8 in, 2 out]
      }
      frame Enabled {
      }
    }
    n363 = Unbundle By Name(w511) -> ("Hatch Retainer States"=w508:T14)
    n364 = case shown="\"Going Down\"" w508 {
      tunnel: [WPI_SolenoidValue."Off" ("Value") WPI_SolenoidValue."On" ("Value") WPI_SolenoidValue."On" ("Value") WPI_SolenoidValue."Off" ("Value")] -> w507
      frame "Fully Down (not retained)", Default {
      }
      frame "Going Up" {
      }
      frame "Fully Up (retained)" {
      }
      frame "Going Down" {
      }
    }
    n365 = call-poly <vilib>:"WPI_SolenoidSet.vi"("Value"=w507, "SolenoidDevRef"=w509) -> ()  [unwired: 8 in, 2 out]
    n366 = disable-structure shown="Enabled" {
      disable-tunnel: [w580 w625] -> w523
      disable-tunnel: w512 -> [w574 w624]
      frame Disabled {
        n367 = disable-structure shown="Enabled" {
          disable-tunnel: [w584 TRUE] -> w577
          disable-tunnel: [w583 TRUE] -> w576
          disable-tunnel: w574 -> [w582 _]
          frame Disabled {
            n368 = Unbundle By Name(w582) -> ("BottomRetainerSwitchDevRef"=w586:T8)
            n369 = Unbundle By Name(w582) -> ("TopRetainerSwitchDevRef"=w588:T8)
            n370 = call <vilib>:"WPI_DigitalInputGetValue.vi"("DigitalInputDevRef"=w588) -> ("Value"=w587:bool)  [unwired: 8 in, 2 out]
            n371 = call <vilib>:"WPI_DigitalInputGetValue.vi"("DigitalInputDevRef"=w586) -> ("Value"=w585:bool)  [unwired: 8 in, 2 out]
            n372 = Not(x=w585) -> (.not. x?=w583:bool)
            n373 = Not(x=w587) -> (.not. x?=w584:bool)
          }
          frame Enabled {
            # "since we aren't using the limit\nswitches now, this acts like they're\nclicked so we don't have to rewrite\neverything"
          }
        }
        n374 = Unbundle By Name(w574) -> ("Hatch Retainer States"=w581:T14)
        n375 = Unbundle By Name(w574) -> ("HatchRetainerMotorDevRef"=w578:T1)
        n376 = Unbundle By Name(w574) -> ("Hatch Retainer Move Up/Down"=w579:bool)
        n377 = case shown="\"Going Down\"" w581 {
          tunnel: [w594 w599 w613 w618] -> w580
          tunnel: w579 -> [w597 _ w614 _]
          tunnel: w577 -> [_ w601 _ _]
          tunnel: w576 -> [_ _ _ w617]
          tunnel: w578 -> [w591 w600 w609 w616]
          tunnel: 0.2 ("Output") -> [_ w598 _ w615]
          frame "Fully Down (not retained)", Default {
            w593 = T33 0 items=["PercentOutput"=0, "Position"=1, "Velocity"=2, "Current"=3, "Follower"=5, "MotionProfile"=6, "MotionMagic"=7, "MotionProfileArc"=10, "Disabled"=15] ("Control Mode")
            n378 = call <vilib>:"CTRE_Phoenix_MotorControl_Set.vi"("Output"=0.0, "Control Mode"=w593, "PhoenixMotorControlDevRef"=w591) -> ()  [unwired: 7 in, 2 out]
            n379 = Select(t=Hatch_Retainer_States."Going Up" ("Hatch Retainer States"), s=w597, f=Hatch_Retainer_States."Fully Down (not retained)" ("Hatch Retainer States")) -> (s? t:f=w594:T14)
          }
          frame "Going Up" {
            n380 = case shown="True" w601 {
              tunnel: w600 -> [w606 _]
              tunnel: [Hatch_Retainer_States."Going Up" ("Hatch Retainer States") Hatch_Retainer_States."Fully Up (retained)" ("Hatch Retainer States")] -> w599
              tunnel: w598 -> [w603 _]
              frame False {
                w604 = T33 0 items=["PercentOutput"=0, "Position"=1, "Velocity"=2, "Current"=3, "Follower"=5, "MotionProfile"=6, "MotionMagic"=7, "MotionProfileArc"=10, "Disabled"=15] ("Control Mode")
                n381 = Negate(x=w603) -> (-x=w602:dbl)
                n382 = call <vilib>:"CTRE_Phoenix_MotorControl_Set.vi"("Output"=w602, "Control Mode"=w604, "PhoenixMotorControlDevRef"=w606) -> ()  [unwired: 7 in, 2 out]
              }
              frame True {
              }
            }
          }
          frame "Fully Up (retained)" {
            w610 = T33 0 items=["PercentOutput"=0, "Position"=1, "Velocity"=2, "Current"=3, "Follower"=5, "MotionProfile"=6, "MotionMagic"=7, "MotionProfileArc"=10, "Disabled"=15] ("Control Mode")
            n383 = call <vilib>:"CTRE_Phoenix_MotorControl_Set.vi"("Output"=0.0, "Control Mode"=w610, "PhoenixMotorControlDevRef"=w609) -> ()  [unwired: 7 in, 2 out]
            n384 = Select(t=Hatch_Retainer_States."Going Down" ("Hatch Retainer States"), s=w614, f=Hatch_Retainer_States."Fully Up (retained)" ("Hatch Retainer States")) -> (s? t:f=w613:T14)
          }
          frame "Going Down" {
            n385 = case shown="True" w617 {
              tunnel: [Hatch_Retainer_States."Going Down" ("Hatch Retainer States") Hatch_Retainer_States."Fully Down (not retained)" ("Hatch Retainer States")] -> w618
              tunnel: w616 -> [w621 _]
              tunnel: w615 -> [w619 _]
              frame False {
                w620 = T33 0 items=["PercentOutput"=0, "Position"=1, "Velocity"=2, "Current"=3, "Follower"=5, "MotionProfile"=6, "MotionMagic"=7, "MotionProfileArc"=10, "Disabled"=15] ("Control Mode")
                n386 = call <vilib>:"CTRE_Phoenix_MotorControl_Set.vi"("Output"=w619, "Control Mode"=w620, "PhoenixMotorControlDevRef"=w621) -> ()  [unwired: 7 in, 2 out]
              }
              frame True {
              }
            }
          }
        }
      }
      frame Enabled {
        n387 = disable-structure shown="Enabled" {
          disable-tunnel: [w634 TRUE] -> w628
          disable-tunnel: [w633 TRUE] -> w627
          disable-tunnel: w624 -> [w632 _]
          frame Disabled {
            n388 = Unbundle By Name(w632) -> ("BottomRetainerSwitchDevRef"=w636:T8)
            n389 = Unbundle By Name(w632) -> ("TopRetainerSwitchDevRef"=w638:T8)
            n390 = call <vilib>:"WPI_DigitalInputGetValue.vi"("DigitalInputDevRef"=w638) -> ("Value"=w637:bool)  [unwired: 8 in, 2 out]
            n391 = call <vilib>:"WPI_DigitalInputGetValue.vi"("DigitalInputDevRef"=w636) -> ("Value"=w635:bool)  [unwired: 8 in, 2 out]
            n392 = Not(x=w635) -> (.not. x?=w633:bool)
            n393 = Not(x=w637) -> (.not. x?=w634:bool)
          }
          frame Enabled {
            # "since we aren't using the limit\nswitches now, this acts like they're\nclicked so we don't have to rewrite\neverything"
          }
        }
        n394 = Unbundle By Name(w624) -> ("Hatch Retainer States"=w631:T14)
        n395 = Unbundle By Name(w624) -> ("HatchRetainerMotorDevRef"=w629:T1)
        n396 = Unbundle By Name(w624) -> ("Hatch Retainer Move Up/Down"=w630:bool)
        n397 = case shown="\"Fully Up (retained)\"" w631 {
          tunnel: [w644 Hatch_Retainer_States."Fully Up (retained)" ("Hatch Retainer States") w654 Hatch_Retainer_States."Fully Down (not retained)" ("Hatch Retainer States")] -> w625
          tunnel: w630 -> [w647 _ w655 _]
          tunnel: w628 -> [_ _ _ _]
          tunnel: w627 -> [_ _ _ _]
          tunnel: w629 -> [w641 _ w650 _]
          tunnel: 0.2 ("Output") -> [_ _ _ _]
          frame "Fully Down (not retained)", Default {
            w643 = T33 0 items=["PercentOutput"=0, "Position"=1, "Velocity"=2, "Current"=3, "Follower"=5, "MotionProfile"=6, "MotionMagic"=7, "MotionProfileArc"=10, "Disabled"=15] ("Control Mode")
            n398 = call <vilib>:"CTRE_Phoenix_MotorControl_Set.vi"("Output"=0.0, "Control Mode"=w643, "PhoenixMotorControlDevRef"=w641) -> ()  [unwired: 7 in, 2 out]
            n399 = Select(t=Hatch_Retainer_States."Going Up" ("Hatch Retainer States"), s=w647, f=Hatch_Retainer_States."Fully Down (not retained)" ("Hatch Retainer States")) -> (s? t:f=w644:T14)
          }
          frame "Going Up" {
            # "no longer need this case since \nwe switched to a pneumatic\nretainer"
          }
          frame "Fully Up (retained)" {
            w651 = T33 0 items=["PercentOutput"=0, "Position"=1, "Velocity"=2, "Current"=3, "Follower"=5, "MotionProfile"=6, "MotionMagic"=7, "MotionProfileArc"=10, "Disabled"=15] ("Control Mode")
            n400 = call <vilib>:"CTRE_Phoenix_MotorControl_Set.vi"("Output"=0.0, "Control Mode"=w651, "PhoenixMotorControlDevRef"=w650) -> ()  [unwired: 7 in, 2 out]
            n401 = Select(t=Hatch_Retainer_States."Going Down" ("Hatch Retainer States"), s=w655, f=Hatch_Retainer_States."Fully Up (retained)" ("Hatch Retainer States")) -> (s? t:f=w654:T14)
          }
          frame "Going Down" {
            # "no longer need this case since \nwe switched to a pneumatic\nretainer"
          }
        }
      }
    }
    n402 = global read "Robot Global Data.vi" "Which Robot?"() -> (w521:T29)
    n403 = global read "Robot Global Data.vi" "Which Robot?"() -> (w520:T29)
    n404 = Unbundle By Name(w512) -> ("Hatch Collector Wanted Angle"=w515:dbl)
    n405 = Unbundle By Name(w512) -> ("Hatch Collector Actual Angle"=w514:dbl)
    n406 = case shown="\"Practice Bot\"" w520 {
      tunnel: [w731 T32 {"proportional gain (Kc)"=0.0, "integral time (Ti, min)"=0.0, "derivative time (Td, min)"=0.0} ("PID gains") T32 {"proportional gain (Kc)"=0.004, "integral time (Ti, min)"=0.0, "derivative time (Td, min)"=0.0} ("PID gains")] -> w519
      frame "Competition Bot", Default {
        # "9.7% motor speed seems\nto be minimum to move"
        n407 = disable-structure shown="Enabled" {
          disable-tunnel: [T32 {"proportional gain (Kc)"=0.03, "integral time (Ti, min)"=0.003, "derivative time (Td, min)"=0.0} ("PID gains") T32 {"proportional gain (Kc)"=0.035, "integral time (Ti, min)"=0.0, "derivative time (Td, min)"=0.0} ("PID gains")] -> w731
          frame Disabled {
          }
          frame Enabled {
          }
        }
      }
      frame "Practice Bot" {
      }
      frame "Code Bot" {
        # "p = 0.008 is WAY too fast"
        # "for code bot:\nwe ended with p = 0.004,\nbut the motor has to turn\nso slowly on the code bot\nthat no PID values would\nreally work well"
      }
    }
    n408 = case shown="\"Competition Bot\", Default" w521 {
      tunnel: [cluster{"output high":dbl, "output low":dbl} {"output high"=0.2, "output low"=-0.4} ("output range") cluster{"output high":dbl, "output low":dbl} {"output high"=0.15, "output low"=-0.15} ("output range") cluster{"output high":dbl, "output low":dbl} {"output high"=0.15, "output low"=-0.15} ("output range")] -> w513
      frame "Competition Bot", Default {
      }
      frame "Practice Bot" {
      }
      frame "Code Bot" {
      }
    }
    n409 = call-poly <vilib>:"PID.vi"("output range"=w513, "PID gains"=w519, "process variable"=w514, "setpoint"=w515) -> ("output"=w543:dbl)  [unwired: 6 in, 1 out]
    n410 = Unbundle By Name(w512) -> ("HatchCollectorMotorDevRef"=w544:T1)
    n411 = call <vilib>:"WPI_MotorControlSetOutput.vi"("Output"=w543, "MotorControlDevRef"=w544) -> ()  [unwired: 7 in, 3 out]
    n412 = Bundle By Name(cluster=w512, "Hatch Retainer States"=w523) -> (w510:T26)
  }
  n413 = while {
    shift-right: [w828] -> _
    shift-left: w48 -> [w858]
    stop <- FALSE stop-if-true
    # "convert from encoder velocity to motor speed...I think"
    # "aux JS is inverted"
    n414 = Unbundle By Name(w858) -> ("DriveJoystickDevRef"=w869:T9)
    n415 = Unbundle By Name(w858) -> ("AuxJoystickDevRef"=w868:T9)
    n416 = Unbundle By Name(w858) -> ("Robot Mode"=w867:T17)
    n417 = call <vilib>:"WPI_JoystickGetValues.vi"("JoystickDevRef"=w868) -> ("Buttons"=w860:bool[], "Axes"=w861:dbl[], "JoystickDevRef"=w862:T9, "POVs"=w859:i16[])  [unwired: 6 in, 1 out]
    n418 = call <vilib>:"WPI_JoystickGetValues.vi"("JoystickDevRef"=w869) -> ("Buttons"=w864:bool[], "Axes"=w866:dbl[], "JoystickDevRef"=w865:T9, "POVs"=w863:i16[])  [unwired: 6 in, 1 out]
    n419 = Wait (ms)(milliseconds to wait=50) -> ()  [unwired: 1 out]
    n420 = case shown="\"Teleop Enabled\"" w867 {
      tunnel: w858 -> [w1043 w1053 w1054 w1055 w1065 w1066 w1067 w1077 w1078]
      tunnel: [w1043 w1044 w1054 w1056 w1065 w1066 w1067 w1068 w1078] -> w841
      tunnel: w866 -> [_ w1052 _ w1063 _ _ _ w1075 _]
      tunnel: w865 -> [_ w1051 _ w1064 _ _ _ w1076 _]
      tunnel: w864 -> [_ w1050 _ w1062 _ _ _ w1074 _]
      tunnel: w863 -> [_ w1049 _ w1061 _ _ _ w1073 _]
      tunnel: w862 -> [_ w1048 _ w1060 _ _ _ w1072 _]
      tunnel: w861 -> [_ w1047 _ w1059 _ _ _ w1071 _]
      tunnel: w860 -> [_ w1046 _ w1058 _ _ _ w1070 _]
      tunnel: w859 -> [_ w1045 _ w1057 _ _ _ w1069 _]
      frame "Autonomous Disabled", Default {
      }
      frame "Autonomous Enabled" {
        n421 = Bundle By Name(cluster=w1053, "DriveJoystickDevRef"=w1051, "Drive Axes"=w1052, "Drive Buttons"=w1050, "Drive POVs"=w1049, "AuxJoystickDevRef"=w1048, "Aux Axes"=w1047, "Aux Buttons"=w1046, "Aux POVs"=w1045) -> (w1044:T27)
      }
      frame "Teleop Disabled" {
      }
      frame "Teleop Enabled" {
        n422 = Bundle By Name(cluster=w1055, "DriveJoystickDevRef"=w1064, "Drive Axes"=w1063, "Drive Buttons"=w1062, "Drive POVs"=w1061, "AuxJoystickDevRef"=w1060, "Aux Axes"=w1059, "Aux Buttons"=w1058, "Aux POVs"=w1057) -> (w1056:T27)
      }
      frame "Disconnected" {
      }
      frame "Finish" {
      }
      frame "Test Disabled" {
      }
      frame "Test Enabled" {
        n423 = Bundle By Name(cluster=w1077, "DriveJoystickDevRef"=w1076, "Drive Axes"=w1075, "Drive Buttons"=w1074, "Drive POVs"=w1073, "AuxJoystickDevRef"=w1072, "Aux Axes"=w1071, "Aux Buttons"=w1070, "Aux POVs"=w1069) -> (w1068:T27)
      }
      frame "Emergency Stopped" {
      }
    }
    n424 = global read "Robot Global Data.vi" "Robot Mode"() -> (w843:T17)
    n425 = Bundle By Name(cluster=w841, "Robot Mode"=w843) -> (w842:T27)
    n426 = disable-structure shown="Enabled" {
      disable-tunnel: w842 -> [w969 w1013]
      disable-tunnel: w841 -> [w968 w1015]
      disable-tunnel: [_ w1000] -> w838
      frame Disabled {
        # "disabled because the RT code would override the instructions of the LT and LB code using separate bundle by names"
        # "controls both \ncylinders together"
        # "controls back cylinders only"
        # "controls front cylinders only"
        n427 = Unbundle By Name(w968) -> ("Aux Button Indexes.RT Button"=w982:i32)
        n428 = Unbundle By Name(w968) -> ("Aux Buttons"=w981:bool[])
        n429 = Unbundle By Name(w968) -> ("Aux Button Indexes.LT Button"=w984:i32)
        n430 = Unbundle By Name(w968) -> ("Front Cylinders Latch"=w977:bool)
        n431 = Unbundle By Name(w968) -> ("Aux Button Indexes.LB Button"=w999:i32)
        n432 = Unbundle By Name(w968) -> ("Aux Buttons"=w985:bool[])
        n433 = Unbundle By Name(w968) -> ("Back Cylinders Latch"=w974:bool)
        n434 = Unbundle By Name(w968) -> ("Aux Buttons"=w998:bool[])
        n435 = Unbundle By Name(w968) -> ("Back Cylinders Latch"=w990:bool)
        n436 = Unbundle By Name(w968) -> ("Front Cylinders Latch"=w993:bool)
        n437 = Index Array(array=w981, index=w982) -> (element=w979:bool)
        n438 = Index Array(array=w985, index=w984) -> (element=w987:bool)
        n439 = Index Array(array=w998, index=w999) -> (element=w996:bool)
        n440 = feedback #10() -> (w980:bool)  [unwired: 1 in]
        n441 = feedback-in #10(w979) -> ()
        n442 = feedback #11() -> (w986:bool)  [unwired: 1 in]
        n443 = feedback-in #11(w987) -> ()
        n444 = feedback #12() -> (w997:bool)  [unwired: 1 in]
        n445 = feedback-in #12(w996) -> ()
        n446 = Greater?(x=w979, y=w980) -> (0:w973:bool)
        n447 = Greater?(x=w987, y=w986) -> (0:w988:bool)
        n448 = Greater?(x=w996, y=w997) -> (0:w995:bool)
        n449 = Not(x=w974) -> (.not. x?=w975:bool)
        n450 = Not(x=w977) -> (.not. x?=w978:bool)
        n451 = Not(x=w990) -> (.not. x?=w989:bool)
        n452 = Not(x=w993) -> (.not. x?=w994:bool)
        n453 = Select(t=w975, s=w973, f=w974) -> (s? t:f=w972:bool)
        n454 = Select(t=w978, s=w973, f=w977) -> (s? t:f=w976:bool)
        n455 = Select(t=w989, s=w988, f=w990) -> (s? t:f=w991:bool)
        n456 = Select(t=w994, s=w995, f=w993) -> (s? t:f=w992:bool)
        n457 = Bundle By Name(cluster=w969, "Front Cylinders Latch"=w992) -> (w983:T27)
        n458 = Bundle By Name(cluster=w983, "Back Cylinders Latch"=w991) -> (w971:T27)
        n459 = Bundle By Name(cluster=w971, "Front Cylinders Latch"=w976) -> (w970:T27)
        n460 = Bundle By Name(cluster=w970, "Back Cylinders Latch"=w972) -> (w967:T27)
      }
      frame Enabled {
        # "controls both \ncylinders together"
        # "controls back cylinders only"
        # "controls front cylinders only"
        n461 = Unbundle By Name(w1015) -> ("Aux Button Indexes.X Button"=w1019:i32)
        n462 = Unbundle By Name(w1015) -> ("Aux Buttons"=w1018:bool[])
        n463 = Unbundle By Name(w1015) -> ("Aux Button Indexes.Y Button"=w1020:i32)
        n464 = Unbundle By Name(w1015) -> ("Aux Buttons"=w1021:bool[])
        n465 = Unbundle By Name(w1015) -> ("Aux Button Indexes.A Button"=w1027:i32)
        n466 = Unbundle By Name(w1015) -> ("Aux Buttons"=w1026:bool[])
        n467 = Unbundle By Name(w1015) -> ("Front Cylinders Latch"=w1006:bool)
        n468 = Unbundle By Name(w1015) -> ("Back Cylinders Latch"=w1003:bool)
        n469 = Index Array(array=w1018, index=w1019) -> (element=w1016:bool)
        n470 = Index Array(array=w1021, index=w1020) -> (element=w1023:bool)
        n471 = Index Array(array=w1026, index=w1027) -> (element=w1024:bool)
        n472 = feedback #13() -> (w1017:bool)  [unwired: 1 in]
        n473 = feedback-in #13(w1016) -> ()
        n474 = feedback #14() -> (w1022:bool)  [unwired: 1 in]
        n475 = feedback-in #14(w1023) -> ()
        n476 = feedback #15() -> (w1025:bool)  [unwired: 1 in]
        n477 = feedback-in #15(w1024) -> ()
        n478 = Greater?(x=w1016, y=w1017) -> (0:w1010:bool)
        n479 = Greater?(x=w1023, y=w1022) -> (0:w1011:bool)
        n480 = Greater?(x=w1024, y=w1025) -> (0:w1012:bool)
        n481 = Or(x=w1012, y=w1010) -> (x .or. y?=w1009:bool)
        n482 = Or(x=w1011, y=w1010) -> (x .or. y?=w1004:bool)
        n483 = Not(x=w1006) -> (.not. x?=w1007:bool)
        n484 = Not(x=w1003) -> (.not. x?=w1005:bool)
        n485 = Select(t=w1007, s=w1009, f=w1006) -> (s? t:f=w1008:bool)
        n486 = Select(t=w1005, s=w1004, f=w1003) -> (s? t:f=w1002:bool)
        n487 = Bundle By Name(cluster=w1013, "Front Cylinders Latch"=w1008) -> (w1014:T27)
        n488 = Bundle By Name(cluster=w1014, "Back Cylinders Latch"=w1002) -> (w1001:T27)
        n489 = disable-structure shown="Disabled" {
          disable-tunnel: w1001 -> [w1032 w1034]
          disable-tunnel: [w1031 w1034] -> w1000
          frame Disabled {
            # "yaw is the angle of our robot\npitch is the angle of elevation of our robot\nroll is how much the robot is rotated about its center"
            n490 = call <vilib>:"Get_YPRHfH.vi"() -> ("YRPHfH"=w1033:T34)  [unwired: 11 in]
            n491 = Unbundle By Name(w1033) -> ("Yaw"=w1030:dbl)
            n492 = Unbundle By Name(w1033) -> ("Pitch"=w1029:dbl)
            n493 = Unbundle By Name(w1033) -> ("Roll"=w1028:dbl)
            n494 = global write "Robot Global Data.vi" "Yaw (clockwise/counter-clockwise)"(w1030) -> ()
            n495 = global write "Robot Global Data.vi" "Roll (forward/backward tipping)"(w1028) -> ()
            n496 = global write "Robot Global Data.vi" "Pitch (left/right tipping)"(w1029) -> ()
            n497 = Bundle By Name(cluster=w1032, "Yaw"=w1030, "Pitch"=w1029, "Roll"=w1028) -> (w1031:T27)
          }
          frame Enabled {
          }
        }
      }
    }
    n498 = Unbundle By Name(w838) -> ("HAB3FrontSolenoidDevRef"=w857:T6)
    n499 = Unbundle By Name(w838) -> ("HABAssisterSolenoidDevRef"=w840:T6)
    n500 = Unbundle By Name(w838) -> ("Front Cylinders Latch"=w834:bool)
    n501 = Unbundle By Name(w838) -> ("HAB3BackSolenoidDevRef"=w851:T6)
    n502 = Unbundle By Name(w838) -> ("Back Cylinders Latch"=w833:bool)
    n503 = disable-structure shown="Disabled" {
      disable-tunnel: w833 -> [w917 _]
      disable-tunnel: w838 -> [w908 _]
      disable-tunnel: [w907 w966] -> w828
      disable-tunnel: w838 -> [w906 w966]
      frame Disabled {
        w924 = T33 2 items=["PercentOutput"=0, "Position"=1, "Velocity"=2, "Current"=3, "Follower"=5, "MotionProfile"=6, "MotionMagic"=7, "MotionProfileArc"=10, "Disabled"=15] ("Control Mode")
        # "would slow down if pos. pitch, \nwhich is opposite of what we want"
        # "base spd +- PID adjustments"
        n504 = Unbundle By Name(w908) -> ("Pitch"=w930:dbl)
        n505 = global read "Robot Global Data.vi" "Which Robot?"() -> (w928:T29)
        n506 = Unbundle By Name(w908) -> ("BkSpdAdjusterMotorDevRef"=w921:T1)
        n507 = Unbundle By Name(w908) -> ("HAB Bk Spd Motor States"=w918:T13)
        n508 = global read "Robot Global Data.vi" "Which Robot?"() -> (w926:T29)
        n509 = case shown="\"Competition Bot\", Default" w926 {
          tunnel: [cluster{"output high":dbl, "output low":dbl} {"output high"=0.2, "output low"=-0.4} ("output range") cluster{"output high":dbl, "output low":dbl} {"output high"=0.15, "output low"=-0.15} ("output range") cluster{"output high":dbl, "output low":dbl} {"output high"=0.15, "output low"=-0.15} ("output range")] -> w925
          frame "Competition Bot", Default {
          }
          frame "Practice Bot" {
          }
          frame "Code Bot" {
          }
        }
        n510 = case shown="\"Code Bot\"" w928 {
          tunnel: [T32 {"proportional gain (Kc)"=0.0, "integral time (Ti, min)"=0.0, "derivative time (Td, min)"=0.0} ("PID gains") T32 {"proportional gain (Kc)"=0.0, "integral time (Ti, min)"=0.0, "derivative time (Td, min)"=0.0} ("PID gains") T32 {"proportional gain (Kc)"=0.0, "integral time (Ti, min)"=0.0, "derivative time (Td, min)"=0.0} ("PID gains")] -> w927
          tunnel: [w960 w962 w964] -> w915
          frame "Competition Bot", Default {
            w960 = 0.0  # Enc. Val at Fully Down
          }
          frame "Practice Bot" {
            w962 = 0.0  # Enc. Val at Fully Down
          }
          frame "Code Bot" {
            w964 = 0.0  # Enc. Val at Fully Down
          }
        }
        n511 = call-poly <vilib>:"PID.vi"("output range"=w925, "PID gains"=w927, "process variable"=w930, "setpoint"=0.0) -> ("output"=w923:dbl)  [unwired: 6 in, 1 out]
        n512 = global read "Robot Global Data.vi" "HAB Bk Spd Encoder Start Value"() -> (w919:dbl)
        n513 = Negate(x=w923) -> (-x=w912:dbl)
        n514 = Add(x=w912, y=0.3) -> (x+y=w913:dbl)
        n515 = call-poly <vilib>:"CTRE_Phoenix_MotorController_Get_Enhanced.vi"("PhoenixMotorControlDevRef"=w921) -> ("Quadrature Position"=w920:i32)  [unwired: 11 in, 3 out]
        n516 = Subtract(x=w920, y=w919) -> (x-y=w909:dbl)
        n517 = Greater Or Equal?(x=w909, y=w915) -> (x >= y?=w914:bool)
        n518 = Less Or Equal To 0?(x=w909) -> (x <= 0?=w910:bool)
        n519 = case shown="\"Fully Up\", Default" w918 {
          tunnel: w917 -> [w934 _ w949 _]
          tunnel: [w935 w936 w945 w951] -> w916
          tunnel: w914 -> [_ w939 _ _]
          tunnel: w913 -> [_ w938 _ _]
          tunnel: [0.0 w937 0.0 w950] -> w911
          tunnel: w910 -> [_ _ _ w952]
          frame "Fully Up", Default {
            n520 = Select(t=HAB_Bk_Spd_Motor_States."Going Down" ("HAB Bk Spd Motor States"), s=w934, f=HAB_Bk_Spd_Motor_States."Fully Up" ("HAB Bk Spd Motor States")) -> (s? t:f=w935:T13)
          }
          frame "Going Down" {
            n521 = case shown="True" w939 {
              tunnel: w938 -> [w941 _]
              tunnel: [w941 0.0] -> w937
              tunnel: [HAB_Bk_Spd_Motor_States."Going Down" ("HAB Bk Spd Motor States") HAB_Bk_Spd_Motor_States."Fully Down" ("HAB Bk Spd Motor States")] -> w936
              frame False {
              }
              frame True {
              }
            }
          }
          frame "Fully Down" {
            n522 = Not(x=w949) -> (.not. x?=w946:bool)
            n523 = Select(t=HAB_Bk_Spd_Motor_States."Going Up" ("HAB Bk Spd Motor States"), s=w946, f=HAB_Bk_Spd_Motor_States."Fully Down" ("HAB Bk Spd Motor States")) -> (s? t:f=w945:T13)
          }
          frame "Going Up" {
            n524 = case shown="True" w952 {
              tunnel: [-0.4 0.0] -> w950
              tunnel: [HAB_Bk_Spd_Motor_States."Going Up" ("HAB Bk Spd Motor States") HAB_Bk_Spd_Motor_States."Fully Up" ("HAB Bk Spd Motor States")] -> w951
              frame False {
                # "gently yeet the \nthing back up, but\nthe velocity don't\nmatter that much"
              }
              frame True {
              }
            }
          }
        }
        n525 = Bundle By Name(cluster=w906, "HAB Bk Spd Motor States"=w916) -> (w907:T27)
        n526 = call <vilib>:"CTRE_Phoenix_MotorControl_Set.vi"("Output"=w911, "Control Mode"=w924, "PhoenixMotorControlDevRef"=w921) -> ()  [unwired: 7 in, 2 out]
      }
      frame Enabled {
      }
    }
    n527 = global write "Robot Global Data.vi" "HAB Back Cylinders Extended?"(w833) -> ()
    n528 = Select(t=WPI_SolenoidValue."On" ("Value"), s=w834, f=WPI_SolenoidValue."Off" ("Value")) -> (s? t:f=w839:T31)
    n529 = global write "Robot Global Data.vi" "HAB Front Cylinders Extended?"(w834) -> ()
    n530 = call-poly <vilib>:"WPI_SolenoidSet.vi"("Value"=w839, "SolenoidDevRef"=w840) -> ()  [unwired: 8 in, 2 out]
    n531 = call-poly <vilib>:"WPI_SolenoidSet.vi"("Value"=w839, "SolenoidDevRef"=w857) -> ()  [unwired: 8 in, 2 out]
    n532 = Select(t=WPI_SolenoidValue."On" ("Value"), s=w833, f=WPI_SolenoidValue."Off" ("Value")) -> (s? t:f=w854:T31)
    n533 = call-poly <vilib>:"WPI_SolenoidSet.vi"("Value"=w854, "SolenoidDevRef"=w851) -> ()  [unwired: 8 in, 2 out]
    n534 = Unbundle By Name(w828) -> ("Aux Button Indexes.B Button"=w830:i32)
    n535 = Unbundle By Name(w828) -> ("Front HAB 3 Limit Switch"=w850:T8)
    n536 = Unbundle By Name(w828) -> ("Back HAB 3 Limit Switch"=w848:T8)
    n537 = Unbundle By Name(w828) -> ("HAB3DriveModuleMotorDevRef"=w849:T1)
    n538 = Unbundle By Name(w828) -> ("Aux Buttons"=w829:bool[])
    n539 = Unbundle By Name(w828) -> ("Aux Axes"=w846:dbl[])
    n540 = Unbundle By Name(w828) -> ("Aux Joystick Indexes.Left Y"=w847:i32)
    n541 = Unbundle By Name(w828) -> ("HAB3DriveModuleMotorDevRef"=w831:T1)
    n542 = global read "Robot Global Data.vi" "Which Robot?"() -> (w835:T29)
    n543 = disable-structure shown="Disabled" {
      disable-tunnel: w828 -> [w1035 _]
      frame Disabled {
        # "maybe use in range and coerce in future to\nprevent drivers from being able to drive\nthe module backwards?"
        # "slows down motor so\nwe don't damage the\ncylinders"
        n544 = Unbundle By Name(w1035) -> ("Aux Joystick Indexes.Right Y"=w1040:i32)
        n545 = Unbundle By Name(w1035) -> ("HAB3DriveModuleMotorDevRef"=w1042:T1)
        n546 = Unbundle By Name(w1035) -> ("Aux Axes"=w1041:dbl[])
        n547 = Index Array(array=w1041, index=w1040) -> (element=w1037:dbl)
        n548 = call "Deadband.vi"("Input"=w1037) -> ("Output"=w1038:dbl)  [unwired: 10 in]
        n549 = Multiply(x=w1038, y=0.3) -> (x*y=w1036:dbl)
        n550 = call <vilib>:"WPI_MotorControlSetOutput.vi"("Output"=w1036, "MotorControlDevRef"=w1042) -> ()  [unwired: 7 in, 3 out]
      }
      frame Enabled {
      }
    }
    n551 = call <vilib>:"WPI_DigitalInputGetValue.vi"("DigitalInputDevRef"=w848) -> ("Value"=w836:bool)  [unwired: 8 in, 2 out]
    n552 = call <vilib>:"WPI_DigitalInputGetValue.vi"("DigitalInputDevRef"=w850) -> ("Value"=w837:bool)  [unwired: 8 in, 2 out]
    n553 = Index Array(array=w846, index=w847) -> (element=w844:dbl)
    n554 = Index Array(array=w829, index=w830) -> (element=w827:bool)
    n555 = case shown="\"Practice Bot\"" w835 {
      tunnel: w837 -> [w899 w903 w905]
      tunnel: [w898 w901 w905] -> w824
      tunnel: [w897 w900 w904] -> w823
      tunnel: w836 -> [w896 w902 w904]
      frame "Competition Bot", Default {
        # "they're \ninverted\nfor some \nreason?"
        n556 = Not(x=w899) -> (.not. x?=w898:bool)
        n557 = Not(x=w896) -> (.not. x?=w897:bool)
      }
      frame "Practice Bot" {
        n558 = Not(x=w903) -> (.not. x?=w901:bool)
        n559 = Not(x=w902) -> (.not. x?=w900:bool)
      }
      frame "Code Bot" {
      }
    }
    n560 = call-poly <vilib>:"CTRE_Phoenix_MotorController_Get_Enhanced.vi"("PhoenixMotorControlDevRef"=w831) -> ("Quadrature Velocity"=w822:i32)  [unwired: 11 in, 3 out]
    n561 = Negate(x=w844) -> (-x=w832:dbl)
    n562 = disable-structure shown="Enabled" {
      disable-tunnel: w822 -> [w874 w875]
      disable-tunnel: [w873 w875] -> w821
      frame Disabled {
        n563 = Divide(x=w874, y=833) -> (x/y=w873:dbl)
      }
      frame Enabled {
      }
    }
    n564 = Or(x=w824, y=w823) -> (x .or. y?=w845:bool)
    n565 = case shown="True" w827 {
      tunnel: w849 -> [w878 w892]
      tunnel: w845 -> [w877 _]
      tunnel: w832 -> [w876 w893]
      frame False {
        n566 = case shown="False" w877 {
          tunnel: w878 -> [w880 w890]
          tunnel: w876 -> [w884 _]
          frame False {
            # "negate the negated JS so it goes forward"
            # "This is a range and coerce. :P \nSees if the joystick is going backwards.\n(If the value is negative).\nIf yes, then output is set to 0.\nIf no, then output is set from the aux\njoystick. \nWe don't want the robot to go \nbackwards off of the platform. LOL"
            # "Slows down the motor output\nso we don't damage the cylinders"
            n567 = call "Deadband.vi"("Input"=w884) -> ("Output"=w888:dbl)  [unwired: 10 in]
            n568 = In Range and Coerce(upper limit=0.0, x=w884, lower limit=-1.0) -> (In Range?=w883:bool)  [unwired: 1 out]
            n569 = Multiply(x=w888, y=0.3) -> (x*y=w879:dbl)
            n570 = Select(t=0.0, s=w883, f=w879) -> (s? t:f=w882:dbl)
            n571 = call <vilib>:"WPI_MotorControlSetOutput.vi"("Output"=w882, "MotorControlDevRef"=w880) -> ()  [unwired: 7 in, 3 out]
          }
          frame True {
            # "If either the \"Front HAB 3 Limit Switch\" or \"Front HAB 3 Limit Switch\"\nis pressed, the HAB 3 Drive Module set output will be \"0.\" \n- Preventing the DRIVER from moving too far forward into\nthe HAB 3 Platform, which can damage the cylinders.\n\nIf not, the aux joysick will control the set output.\n- Enabling the DRIVER to drive forward until the robot reaches the\nplatform"
            n572 = call <vilib>:"WPI_MotorControlSetOutput.vi"("Output"=0.0, "MotorControlDevRef"=w890) -> ()  [unwired: 7 in, 3 out]
          }
        }
      }
      frame True {
        # "if da B button is pressed, then\nit overrides the switches and\nallows the HAB Drive Mod to \ngo forward. :D!!"
        # "negate the negated JS so it goes forward"
        # "This is a range and coerce. :P \nSees if the joystick is going backwards.\n(If the value is negative).\nIf yes, then output is set to 0.\nIf no, then output is set from the aux\njoystick. \nWe don't want the robot to go \nbackwards off of the platform. LOL"
        # "Slows down the motor output\nso we don't damage the cylinders"
        n573 = call "Deadband.vi"("Input"=w893) -> ("Output"=w895:dbl)  [unwired: 10 in]
        n574 = Multiply(x=w895, y=0.3) -> (x*y=w891:dbl)
        n575 = call <vilib>:"WPI_MotorControlSetOutput.vi"("Output"=w891, "MotorControlDevRef"=w892) -> ()  [unwired: 7 in, 3 out]
      }
    }
    n576 = global write "Robot Global Data.vi" "HAB Module Actual Velocity"(w821) -> ()
    n577 = call-poly <vilib>:"NT Write Value.vi"("Boolean"=w824, "Name"="Front HAB 3 Limit Switch") -> ()  [unwired: 9 in, 1 out]
    n578 = call-poly <vilib>:"NT Write Value.vi"("Boolean"=w823, "Name"="Back HAB 3 Limit Switch") -> ()  [unwired: 9 in, 1 out]
  }
  n579 = disable-structure shown="Enabled" {
    frame Disabled {
      # "collector \nangle \nup/down"
      # "HAB 3 drive\nmodule"
      # "RJ"
      # "LJ"
      # "angle preset hover\nfor dust pan"
      # "angle preset out/down"
      # "angle preset in/up"
      # "lift hatch"
      # "retain hatch"
      # "kick hatch"
      # "RB"
      # "RT"
      # "LB"
      # "LT"
      # "back cylinders only"
      # "both cylinders"
      # "front cylinders only"
      # "x"
      # "a"
      # "b"
      # "y"
    }
    frame Disabled {
      # "inaccurate"
      # "collector \nangle \nup/down."
      # "HAB 3 drive\nmodule."
      # "RJ"
      # "LJ"
      # "angle preset hover\nfor dust pan."
      # "angle preset out/down"
      # "angle preset in/up."
      # "lift hatch."
      # "retain hatch."
      # "kick hatch."
      # "RB"
      # "RT"
      # "LB"
      # "LT"
      # "back cylinders only."
      # "both cylinders."
      # "front cylinders only."
      # "x"
      # "a"
      # "b"
      # "y"
    }
    frame Enabled {
    }
  }
  n580 = call "Reset Drive Encoders.vi"() -> ()  [unwired: 12 in]
  "error out" <- "error in"
